vi "StandAlone_TransientDataCollection_Overhaul.vi"(8 "error in":errorcluster, 11 "Oscilloscope Configuration Array":T2(array[cluster]) {"vertical coupling" items=["AC", "DC", "Ground"]}) -> (0 "error out":errorcluster)   [LabVIEW 2019]
uses:
  <instrlib>/niScope/Controls/niScope vertical coupling.ctl
  <vilib>/Utility/file.llb/Write Delimited Spreadsheet (string).vi
  <instrlib>/niScope/Configure/Trigger/niScope Configure Trigger Software.vi
  <instrlib>/niScope/Acquire/Fetch/niScope Multi Fetch Binary 16.vi
panel:
  out "Sample Rate IND 2":dbl
  in  "stop 2":bool
  in  "Plot Data?":bool
  in  "numSamples":i32=-1
  in  "ON/OFF":bool
  in  "Using an RF Source?":bool
  in  "power (dBm)":dbl
  in  "frequency (GHz)":dbl
  in  "Apply RF Source Changes":bool
  in  "RF Source":refnum<visa-resource-name>
  out "current limit ind":dbl
  out "Channel 0 Reference Values":dbl[](array[numeric])
  out "CHANNEL 7 NAME":string
  out "CHANNEL 6 NAME":string
  out "CHANNEL 5 NAME":string
  out "CHANNEL 4 NAME":string
  out "CHANNEL 3 NAME":string
  out "CHANNEL 2 NAME":string
  out "CHANNEL 1 NAME":string
  out "CHANNEL 0 NAME":string
  out "RUN_FOLDER":path
  out "RESTART PROGRAM SOON (DATACOLLECT)":bool
  out "Sample Rate IND":dbl
  out "Channel To Mitigate (0-7) IND":i32
  out "Collecting Data":bool
  out "RESTART PROGRAM SOON (DATASTORE)":bool
  out "Threshold Value":dbl
  out "Num Loop 4 Reset Graph":i32
  out "Channel Graph Cumulative 7":dbl[](graph)
  out "Channel Graph Cumulative 6":dbl[](graph)
  out "Channel Graph Cumulative 5":dbl[](graph)
  out "Channel Graph Cumulative 4":dbl[](graph)
  out "Channel Graph Cumulative 3":dbl[](graph)
  out "Channel Graph Cumulative 2":dbl[](graph)
  out "Channel Graph Cumulative 1":dbl[](graph)
  out "Channel Graph Cumulative 0":dbl[](graph)
  out "Channel Graph 7":dbl[](graph)
  out "Channel Graph 6":dbl[](graph)
  out "Channel Graph 5":dbl[](graph)
  out "Channel Graph 4":dbl[](graph)
  out "Channel Graph 3":dbl[](graph)
  out "Channel Graph 2":dbl[](graph)
  out "Channel Graph 1":dbl[](graph)
  out "Channel Graph 0":dbl[](graph)
  in  "Channel To Mitigate (0-7)":i32
  out "Last Point Fetched":i32
  out "Total Points Fetched":i32
  out "NUMBER SAMPLES":i32
  out "XINC":dbl
  out "Nominal Current IND":dbl
  out "Percent Threshold IND":dbl
  out "EXCEED THRESHOLD":bool
  out "EXCEED DURATION":bool
  out "Over Threshold Number":i32
  out "number of resets":i32
  out "ENABLE STATE":bool
  in  "DC Power On":bool
  in  "TRANSIENT TIME DURATION (ms)":dbl=500.0
  in  "milliseconds to wait":u32
  in  "vertical coupling":T1=1 items=["AC", "DC", "Ground"]
  in  "min record length":i32=100000
  in  "INTIALIZE SCOPE":bool
  in  "50 ohm vertical range (V)":dbl=10.0 caption="50 ohm vertical range" format="%.2f"
  in  "Channel 0 50 ohms?":bool
  out "wfm info IND":T3(array[cluster]) caption="wfm info" {"reserved2" format="%.2f"; "reserved1" format="%.2f"; "offset" format="%^.3e"; "gain" format="%^.3e"; "xIncrement" format="%^.3e"; "relativeInitialX" format="%^.3e"; "absoluteInitialX" format="%^.3e"}
  out "AUTOMITIGATION ENABLED IND":bool
  in  "AUTOMITIGATION ENABLED":bool
  out "Vertical Range (V) IND":dbl=30.0 caption="Vertical Range (V)" format="%_3g"
  out "channels IND":string="0" caption="channels"
  out "Min. Sample Rate IND":dbl=50000.0 caption="Min. Sample Rate" format="%#_6p"
  in  "Ion (ex. Kr)":string
  in  "Effective LET":string
  in  "Board Number":string
  in  "DUT":string
  in  "Beam On?":bool
  in  "Percent Threshold":dbl
  in  "Nominal Mitigation Value":dbl
  out "Number Of Channels":i32
  in  "Plot Data?":bool=TRUE
  out "CURRENTPATH":path
  out "FOLDERCREATED":bool=TRUE
  out "IndicatorOutputs":cluster{"Run Information":string, string}
  out "Latchup_or_Transient":bool
  out "BinaryRefObjects":T4
  out "OscopeParamPath":path
  out "INITIALIZED":bool
  in  "APPLYPATH":bool
  in  "INPUTPATH":path=path "C:/Campaigns/LBNL_May_2025"
  in  "Max Points per Fetch":i32=-1
  in  "channels":string="Current,Vin,Vout1,Vout2,PowerGood1_2,EN1,EN2,BeamSignal" caption="channels (comma separated)"
  in  "Oscilloscope":refnum<k15>="PXIe-5172"
  in  "Min. Sample Rate":dbl=50000.0 format="%#_6p"
  in  "Vertical Range (V)":dbl=30.0 format="%_3g"
  out "RECORDING DATA":bool
  in  "BEGIN RECORDING":bool
  out "Present Mitigation Information":string
  out "NIDCPOWER_VOLT_CONF":dbl caption="voltage level IND" format="%.6p"
  out "NIDCPOWER_CHAN_CONF":string
  in  "NIDCPOWER_VOLT":dbl caption="voltage level" format="%.6p"
  in  "NIDCPOWER_CHAN":string="0"
  in  "resource name":refnum<k15>="Slot_4_PXIe4139" caption="DC Power PSU"
  in  "CHANGE MITIGATION":bool
  in  "Mitigation":u16(ring) items=["None", "Hardware", "PowerCycle", "EnableCircuit"]
  out "FINISH PROGRAM":bool
  in  "FORCED RESET":bool
  out "POWER STATE":bool
  in  "Channels to Parallelize (if selected)":u16(ring) items=["I1+I2", "ALL", "I2+I3"]
  out "Present Channel Configuration":string
  out "Channels Configured and Values":string[][](array[string])
  in  "Combination":u16(ring) items=["OFF", "SERIES", "PARALLEL"]
  in  "PSU":refnum<visa-resource-name>="USB0::0x05E6::0x2230::802901012767010005::INSTR"
  in  "Current Limit Channel 3":dbl
  in  "Current Limit Channel 2":dbl
  in  "Current Limit Channel 1":dbl
  in  "Voltage Channel 3":dbl
  in  "Voltage Channel 2":dbl
  in  "Voltage Channel 1":dbl
  in  "stop":bool
  in  "APPLY POWER SETTINGS":bool
  in  "POWER ON":bool
  # "11 In order, name all of the channels 0-7"
  # "3 press the white arrow"
  # "10 this is the maximum. Make it smaller for better resolution"
  # "OSCILLOSCOPE BLOCK"
  # "DATA BLOCK"
  # "5 enter where the data"
  # "Use this for step three"
  # "9 if needed"
  # "12 set the scope to the configurations from steps 9-11 on device"
  # "Nothing behind here"
  # "6 enter in values before each run"
  # "need to fix this"
  # "13,16 begin recording data"
  # "1"
  # "17 end program"
  # "2"
  # "14,15 saying the beam is on or could just have the TTL logic"
  # "7 enter in values before each run"
  # "POWER BLOCK"
  # "NI DCPower"
  # "NOTE THAT VISA POWER HAS THE NI DC POWER TURN OFF AS WELL"
  # "4"
  # "Current"
  # "8 power on device"
  # "Ignore all of this"
  # "7 power on device"
  # "7 power on device"
  # "7 power on device"
  # "7 power on device"
  # "7 power on device"
  # "7 power on device"
  # "7 power on device"
  # "7 power on device"
  # "7 power on device"
  # "7 power on device"
  # "7 power on device"
  # "7 power on device"
types:
  T1 = typedef "niScope vertical coupling.ctl" = i32
  T2 = cluster{"instrument handle out":refnum<k15>, string[], string[], "vertical range":dbl, "vertical coupling":T1, "Channel 0 50 ohms?":bool, "50 ohm vertical range (V)":dbl, "min record length":i32, "Actual Sample Rate":dbl, "channel names list":string}[]
  T3 = cluster{"actualSamples":i32, "absoluteInitialX":dbl, "relativeInitialX":dbl, "xIncrement":dbl, "offset":dbl, "gain":dbl, "reserved1":dbl, "reserved2":dbl}[]
  T4 = cluster{"appended path":path, "refnum out":refnum<file>, "refnum out":refnum<file>, "refnum out":refnum<file>}
  T5 = cluster{dbl[], dbl[], dbl[], dbl[], dbl[], dbl[], dbl[], dbl[]}
  T6 = cluster{"instrument handle out":refnum<k15>, string[], string[], "vertical range":dbl, "vertical coupling":T1, "Channel 0 50 ohms?":bool, "50 ohm vertical range (V)":dbl, "min record length":i32, "Actual Sample Rate":dbl, "channel names list":string}
  T7 = cluster{"array":dbl[], "array":dbl[], "array":dbl[], "array":dbl[], "array":dbl[], "array":dbl[], "array":dbl[], "array":dbl[]}
  T8 = cluster{"wfm info":cluster{"actualSamples":i32, "absoluteInitialX":dbl, "relativeInitialX":dbl, "xIncrement":dbl, "offset":dbl, "gain":dbl, "reserved1":dbl, "reserved2":dbl}[], "wfm":i16[][], "Beam On?":bool, i32}
  T9 = enum16{"open", "replace", "create", "open or create", "replace or create", "replace or create with confirmation"}
  T10 = enum16{"big-endian, network order", "native, host order", "little-endian"}
  T11 = cluster{"wfm info":cluster{"actualSamples":i32, "absoluteInitialX":dbl, "relativeInitialX":dbl, "xIncrement":dbl, "offset":dbl, "gain":dbl, "reserved1":dbl, "reserved2":dbl}[], "wfm":i16[][]}
  T12 = cluster{"actualSamples":i32, "absoluteInitialX":dbl, "relativeInitialX":dbl, "xIncrement":dbl, "offset":dbl, "gain":dbl, "reserved1":dbl, "reserved2":dbl}
  T13 = cluster{"AUTOMITIGATION ENABLED IND":bool, "Present Mitigation Information":string}
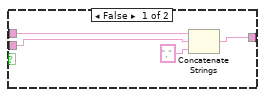
[diagram p2: hidden frame]
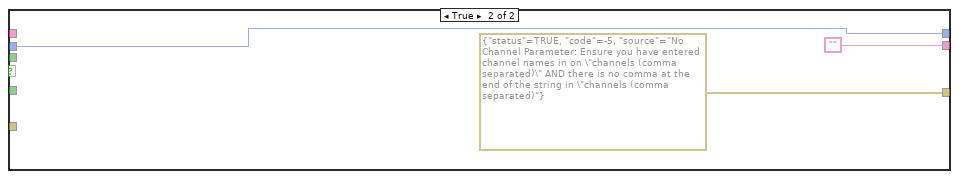
[diagram p3: hidden frame]
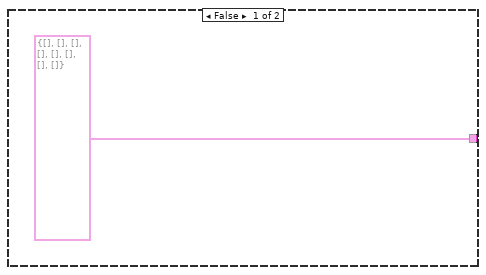
[diagram p6: hidden frame]
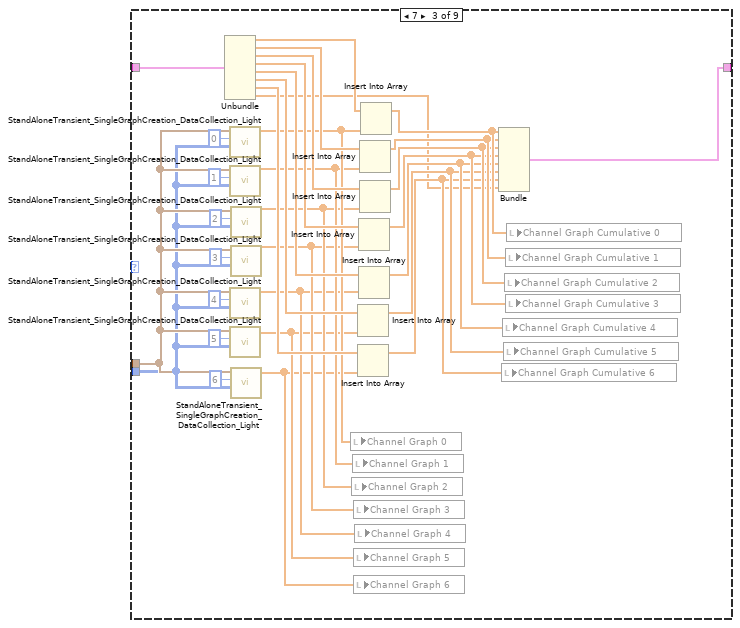
[diagram p8: hidden frame]
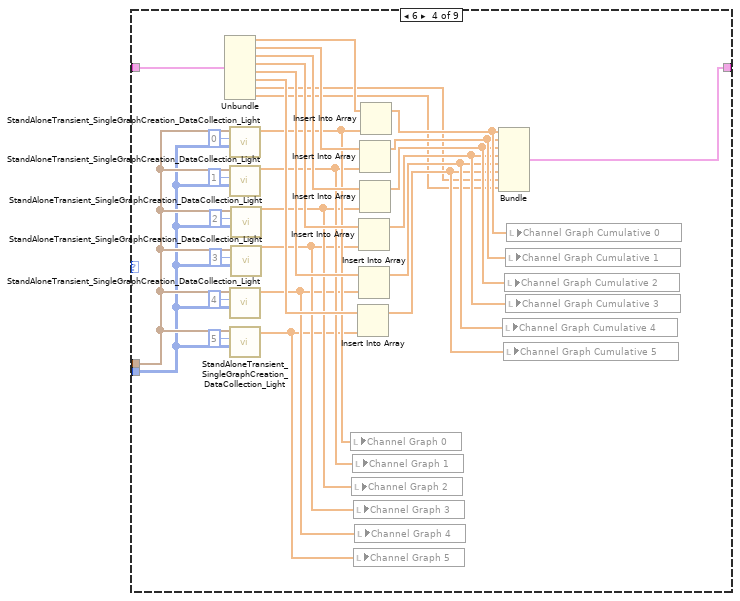
[diagram p9: hidden frame]
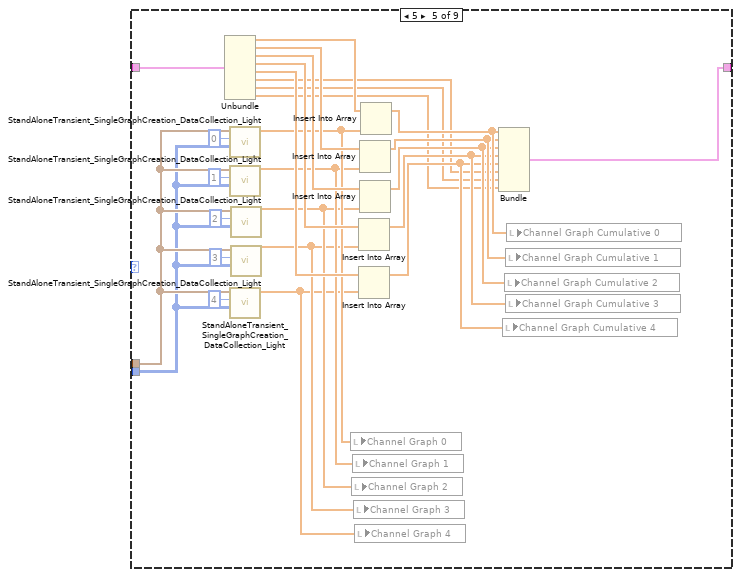
[diagram p10: hidden frame]
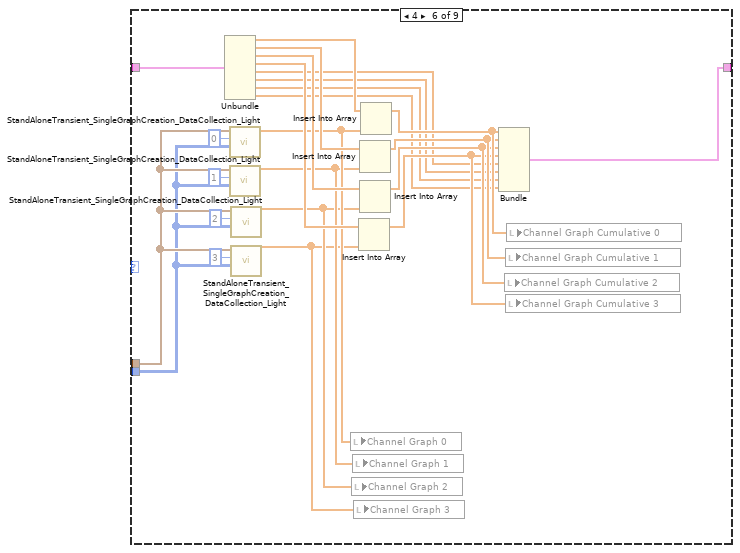
[diagram p11: hidden frame]
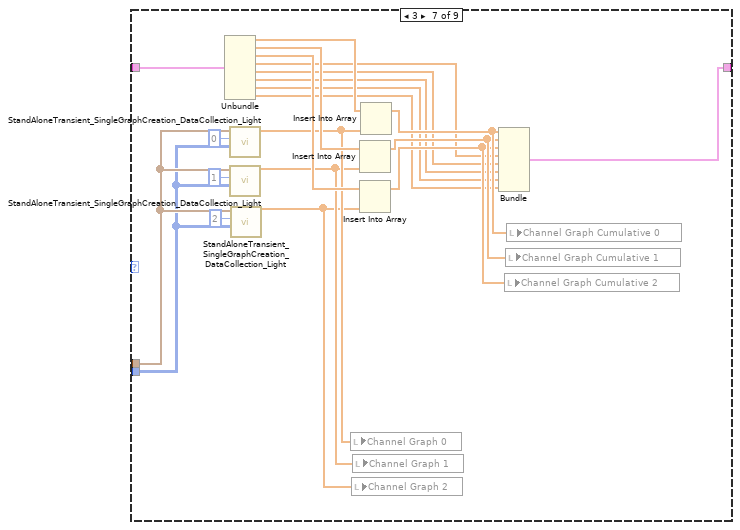
[diagram p12: hidden frame]
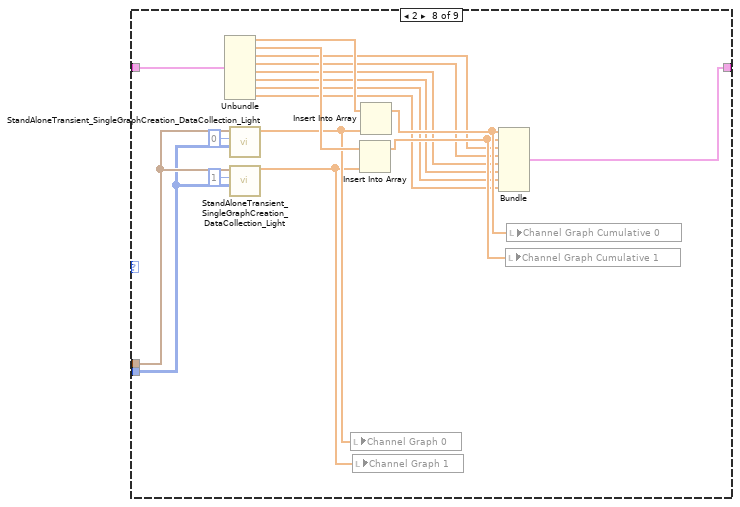
[diagram p13: hidden frame]
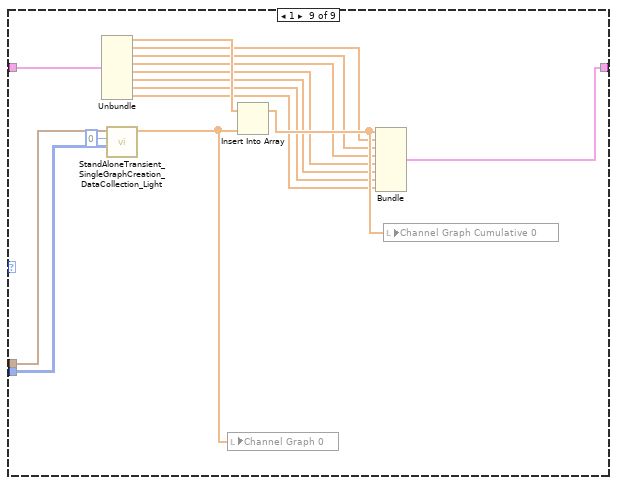
[diagram p14: hidden frame]
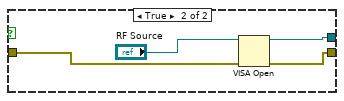
[diagram p16: hidden frame]
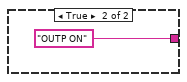
[diagram p18: hidden frame]
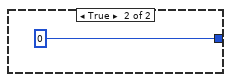
[diagram p19: hidden frame]
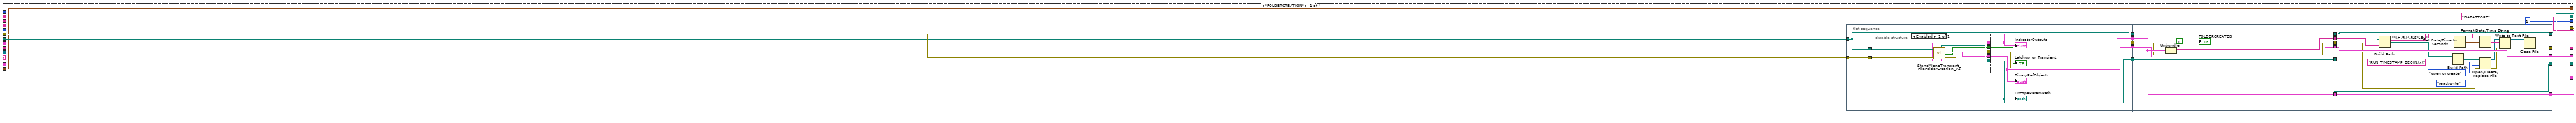
[diagram p20: hidden frame]
diagram:
  n1 = disable-structure shown="Disabled" {
    frame Disabled {
      n2 = Index Array(array="Oscilloscope Configuration Array", index=0) -> (element=w13:T6)
      n3 = Unbundle(w13) -> ("instrument handle out"=w7:refnum<k15>, w10:string[], "channel names list"=w12:string)  [unwired: 7 out]
      n4 = Array Size(array=w10) -> (size(s)=w9:i32)
      n5 = call <instrlib>:"niScope Initiate Acquisition.vi"("instrument handle"=w7, "error in"="error in") -> ("instrument handle out"=w5:refnum<k15>, "error out"=w6:errorcluster)  [unwired: 12 in]
      n6 = disable-structure shown="Disabled" {
        frame Disabled {
          n7 = flat-sequence {
            tunnel: _ -> [w29]
            tunnel: _ -> [w30]
            tunnel: _ -> [w31]
            tunnel: _ -> [w26]
            tunnel: _ -> [w32]
            tunnel: _ -> [w24]
            tunnel: _ -> [w33]
            tunnel: [w33] -> w22
            tunnel: [w23] -> w21
            tunnel: [w32] -> w20
            tunnel: [w25] -> w19
            tunnel: [w31] -> w18
            tunnel: [w30] -> w17
            tunnel: [w29] -> w16
            tunnel: [w118] -> _
            tunnel: [w117] -> _
            tunnel: ["WAIT4FOLDER"] -> _
            tunnel: _ -> [w100]
            tunnel: _ -> [w93]
            tunnel: [w91] -> _
            tunnel: w22 -> [w116]
            tunnel: w21 -> [w115]
            tunnel: w20 -> [w114]
            tunnel: w19 -> [w90]
            tunnel: w18 -> [w99]
            tunnel: w17 -> [w98]
            tunnel: w16 -> [w92]
            tunnel: [w90] -> _
            frame #0 {
              n8 = while {
                shift-right: [w49] -> _
                shift-left: w26 -> [w50]
                shift-right: [w35] -> _
                shift-left: 0 -> [w41]
                shift-right: [w43] -> w25
                shift-left: "" -> [w39]
                tunnel: [w49] -> _ mode=indexing
                tunnel: w24 -> [w38]
                tunnel: [w37] -> w23
                i -> [w48]
                stop <- w47 stop-if-true
                n9 = flat-sequence {
                  tunnel: w50 -> [w60]
                  tunnel: w48 -> [_]
                  tunnel: [w58] -> w46
                  tunnel: [w51] -> w45
                  tunnel: [w52] -> w44
                  tunnel: [w57] -> w42
                  tunnel: w41 -> [w57]
                  tunnel: [w56] -> w40
                  tunnel: w39 -> [w56]
                  tunnel: [w51] -> w34
                  tunnel: w46 -> [w72]
                  tunnel: w45 -> [w63]
                  tunnel: w44 -> [w71]
                  tunnel: w42 -> [w69]
                  tunnel: w40 -> [w68]
                  tunnel: w38 -> [w67]
                  tunnel: [w72] -> w49
                  tunnel: [w63] -> w47
                  tunnel: [w70] -> w43
                  tunnel: [w66] -> w37
                  tunnel: [w65] -> w36
                  tunnel: w34 -> [w64]
                  frame #0 {
                    n10 = Match Pattern(string=w60, regular expression=",") -> (before substring=w55:string, after substring=w58:string, offset past match=w62:i32)  [unwired: 1 in, 1 out]
                    n11 = Equal?(x=w55, y="") -> (x = y?=w53:bool)
                    n12 = Equal?(x=w62, y=-1) -> (x = y?=w51:bool)
                    n13 = And(x=w51, y=w53) -> (x .and. y?=w52:bool)
                  }
                  frame #1 {
                    n14 = case shown="False" w71 {
                      tunnel: [w73 ""] -> w70
                      tunnel: w69 -> [w78 w87]
                      tunnel: w68 -> [w76 _]
                      tunnel: [w78 w87] -> w65
                      tunnel: w67 -> [w77 _]
                      tunnel: [w77 errorcluster {"status"=TRUE, "code"=-5, "source"="No Channel Parameter: Ensure you have entered channel names in on \"channels (comma separated)\" AND there is no comma at the end of the string in \"channels (comma separated)"} ("error out")] -> w66
                      tunnel: w64 -> [_ _]
                      tunnel: w63 -> [w74 _]
                      frame False {
                        n15 = Number To Decimal String(number=w78) -> (decimal integer string=w75:string)  [unwired: 1 in]
                        n16 = case shown="True" w74 {
                          tunnel: w76 -> [w82 w85]
                          tunnel: w75 -> [w81 w84]
                          tunnel: [w79 w83] -> w73
                          frame False {
                            n17 = Concatenate Strings(w82, w81, "," ("string")) -> (w79:string)
                          }
                          frame True {
                            n18 = Concatenate Strings(w85, w84) -> (w83:string)
                          }
                        }
                      }
                      frame True {
                      }
                    }
                  }
                }
                n19 = Increment(x=w36) -> (x+1=w35:i32)
              }
            }
            frame #1 {
              w119 = u32 0 items=["1 mega ohm"=0, "50 ohms"=2] ("input impedance")
              w124 = 388 items=["Start"=482, "Trigger"=483, "Pretrigger"=477, "Now"=481, "Read Pointer"=388] ("Fetch:Fetch Relative To")
              # "3"
              n20 = String Length(string=w90) -> (length=w112:i32)
              n21 = Match Pattern(string=w90, regular expression="0") -> (offset past match=w102:i32)  [unwired: 1 in, 3 out]
              n22 = call <instrlib>:"niScope Configure Vertical.vi"("instrument handle"=w116, "vertical coupling"=w98, "channels"=w90, "vertical range"=w114, "error in"=w115) -> ("instrument handle out"=w121:refnum<k15>, "error out"=w120:errorcluster)  [unwired: 9 in]
              n23 = Quotient & Remainder(x=w112, y=2) -> (x-y*floor(x/y)=w109:i32, floor(x/y)=w110:i32)
              n24 = Not Equal?(x=w102, y=-1) -> (x != y?=w103:bool)
              n25 = And(x=w99, y=w103) -> (x .and. y?=w104:bool)
              n26 = Add(x=w109, y=w110) -> (x+y=w91:i32)
              n27 = call <instrlib>:"niScope Configure Chan Characteristics.vi"("instrument handle"=w121, "channels"=w90, "input impedance"=w119, "maximum input frequency"=0.0, "error in"=w120) -> ("instrument handle out"=w107:refnum<k15>, "error out"=w106:errorcluster)  [unwired: 9 in]
              n28 = case shown="True" w104 {
                tunnel: [w128 w138] -> w97
                tunnel: [w127 w137] -> w96
                tunnel: w107 -> [w128 w132]
                tunnel: w106 -> [w127 w131]
                tunnel: w100 -> [_ w129]
                frame False {
                }
                frame True {
                  w135 = u32 2 items=["1 mega ohm"=0, "50 ohms"=2] ("input impedance")
                  w130 = "0" ("channels")
                  n29 = call <instrlib>:"niScope Configure Vertical.vi"("instrument handle"=w132, "channels"=w130, "vertical range"=w129, "error in"=w131) -> ("instrument handle out"=w134:refnum<k15>, "error out"=w133:errorcluster)  [unwired: 10 in]
                  n30 = call <instrlib>:"niScope Configure Chan Characteristics.vi"("instrument handle"=w134, "channels"=w130, "input impedance"=w135, "maximum input frequency"=0.0, "error in"=w133) -> ("instrument handle out"=w138:refnum<k15>, "error out"=w137:errorcluster)  [unwired: 9 in]
                }
              }
              n31 = call <instrlib>:"niScope Configure Horizontal Timing.vi"("instrument handle"=w97, "min sample rate"=w92, "error in"=w96, "min record length"=w93) -> ("instrument handle out"=w94:refnum<k15>, "error out"=w95:errorcluster)  [unwired: 10 in]
              n32 = call-poly <instrlib>:"niScope Configure Trigger (poly).vi"("instrument handle"=w94, "error in"=w95) -> ("instrument handle out"=w123:refnum<k15>, "error out"=w122:errorcluster)  [unwired: 12 in]
              n33 = call <instrlib>:"niScope Initiate Acquisition.vi"("instrument handle"=w123, "error in"=w122) -> ("instrument handle out"=w125:refnum<k15>, "error out"=w126:errorcluster)  [unwired: 12 in]
              n34 = property class="niScope" props=["Fetch:Fetch Relative To", "Acquisition:Binary Sample Width", "Actual Sample Rate", "Actual Record Length"](reference=w125, error in=w126, "Fetch:Fetch Relative To"=w124) -> (reference out=w118:refnum<k15>, error out=w117:errorcluster, "Actual Sample Rate"=→"Sample Rate IND 2":dbl)  [unwired: 2 out]
            }
          }
        }
        frame Enabled {
        }
      }
      n35 = while {
        shift-right: [w148] -> w4
        shift-left: w6 -> [w158]
        tunnel: w5 -> [w157]
        tunnel: w12 -> [w156]
        tunnel: "numSamples" -> [w155]
        tunnel: w9 -> [w154]
        shift-right: [w151] -> _
        shift-left: _ -> [w150]
        tunnel: [w146] -> w3
        shift-right: [w139] -> _
        shift-left: 0 -> [w142]
        stop <- w147 stop-if-true
        n36 = Increment(x=w142) -> (x+1=w139:i32)
        n37 = Greater?(x=w139, y=1000000) -> (0:w143:bool)
        n38 = Not(x=w143) -> (.not. x?=w145:bool)
        n39 = call-poly <instrlib>:"niScope Fetch (poly).vi"("timeout"=0.0, "error in"=w158, "numSamples"=w155, "channels"=w156, "instrument handle"=w157) -> ("error out"=w148:errorcluster, "wfm"=w152:i16[][], "wfm info"=w153:T3, "instrument handle out"=w146:refnum<k15>)  [unwired: 3 in]
        n40 = Or(x="Plot Data?", y=w145) -> (x .or. y?=w140:bool)
        n41 = case shown="True" w140 {
          tunnel: w154 -> [_ w165]
          tunnel: w153 -> [_ w164]
          tunnel: w152 -> [_ w163]
          tunnel: [T5 {[], [], [], [], [], [], [], []} w162] -> w151
          tunnel: w150 -> [_ w161]
          frame False {
          }
          frame True {
            n42 = case shown="8" w165 {
              tunnel: w164 -> [_ w201 w234 w264 w291 w315 w336 w354 w369]
              tunnel: w163 -> [_ w200 w233 w263 w290 w314 w335 w353 w368]
              tunnel: [w166 w192 w203 w237 w266 w293 w318 w340 w359] -> w162
              tunnel: w161 -> [w166 w191 w226 w257 w285 w310 w332 w351 w367]
              frame 0, Default {
              }
              frame 8 {
                n43 = Unbundle(w191) -> (w183:dbl[], w184:dbl[], w185:dbl[], w186:dbl[], w187:dbl[], w188:dbl[], w189:dbl[], w190:dbl[])
                n44 = call "StandAloneTransient_SingleGraphCreation_DataCollection_Light.vi"("wfm"=w200, "index"=0, "wfm info"=w201) -> ("Array"=w182:dbl[])  [unwired: 8 in]
                n45 = call "StandAloneTransient_SingleGraphCreation_DataCollection_Light.vi"("wfm"=w200, "index"=1, "wfm info"=w201) -> ("Array"=w181:dbl[])  [unwired: 8 in]
                n46 = call "StandAloneTransient_SingleGraphCreation_DataCollection_Light.vi"("wfm"=w200, "index"=4, "wfm info"=w201) -> ("Array"=w178:dbl[])  [unwired: 8 in]
                n47 = call "StandAloneTransient_SingleGraphCreation_DataCollection_Light.vi"("wfm"=w200, "index"=5, "wfm info"=w201) -> ("Array"=w177:dbl[])  [unwired: 8 in]
                n48 = call "StandAloneTransient_SingleGraphCreation_DataCollection_Light.vi"("wfm"=w200, "index"=2, "wfm info"=w201) -> ("Array"=w180:dbl[])  [unwired: 8 in]
                n49 = call "StandAloneTransient_SingleGraphCreation_DataCollection_Light.vi"("wfm"=w200, "index"=3, "wfm info"=w201) -> ("Array"=w179:dbl[])  [unwired: 8 in]
                n50 = call "StandAloneTransient_SingleGraphCreation_DataCollection_Light.vi"("wfm"=w200, "index"=6, "wfm info"=w201) -> ("Array"=w176:dbl[])  [unwired: 8 in]
                n51 = call "StandAloneTransient_SingleGraphCreation_DataCollection_Light.vi"("wfm"=w200, "index"=7, "wfm info"=w201) -> ("Array"=w175:dbl[])  [unwired: 8 in]
                n52 = local write "Channel Graph 0"(w182) -> ()
                n53 = local write "Channel Graph 2"(w180) -> ()
                n54 = local write "Channel Graph 1"(w181) -> ()
                n55 = local write "Channel Graph 3"(w179) -> ()
                n56 = local write "Channel Graph 5"(w177) -> ()
                n57 = local write "Channel Graph 6"(w176) -> ()
                n58 = local write "Channel Graph 7"(w175) -> ()
                n59 = local write "Channel Graph 4"(w178) -> ()
                n60 = Insert Into Array(array=w190, new element=w175) -> (w167:dbl[])  [unwired: 1 in]
                n61 = Insert Into Array(array=w188, new element=w177) -> (w169:dbl[])  [unwired: 1 in]
                n62 = Insert Into Array(array=w189, new element=w176) -> (w168:dbl[])  [unwired: 1 in]
                n63 = Insert Into Array(array=w186, new element=w179) -> (w171:dbl[])  [unwired: 1 in]
                n64 = Insert Into Array(array=w187, new element=w178) -> (w170:dbl[])  [unwired: 1 in]
                n65 = Insert Into Array(array=w184, new element=w181) -> (w173:dbl[])  [unwired: 1 in]
                n66 = Insert Into Array(array=w185, new element=w180) -> (w172:dbl[])  [unwired: 1 in]
                n67 = Insert Into Array(array=w183, new element=w182) -> (w174:dbl[])  [unwired: 1 in]
                n68 = Bundle(w174, w173, w172, w171, w170, w169, w168, w167) -> (w192:T5)  [unwired: 1 in]
                n69 = local write "Channel Graph Cumulative 6"(w168) -> ()
                n70 = local write "Channel Graph Cumulative 4"(w170) -> ()
                n71 = local write "Channel Graph Cumulative 5"(w169) -> ()
                n72 = local write "Channel Graph Cumulative 7"(w167) -> ()
                n73 = local write "Channel Graph Cumulative 2"(w172) -> ()
                n74 = local write "Channel Graph Cumulative 1"(w173) -> ()
                n75 = local write "Channel Graph Cumulative 3"(w171) -> ()
                n76 = local write "Channel Graph Cumulative 0"(w174) -> ()
              }
              frame 7 {
                n77 = Unbundle(w226) -> (w219:dbl[], w220:dbl[], w221:dbl[], w222:dbl[], w223:dbl[], w224:dbl[], w225:dbl[], w204:dbl[])
                n78 = call "StandAloneTransient_SingleGraphCreation_DataCollection_Light.vi"("wfm"=w233, "index"=0, "wfm info"=w234) -> ("Array"=w218:dbl[])  [unwired: 8 in]
                n79 = call "StandAloneTransient_SingleGraphCreation_DataCollection_Light.vi"("wfm"=w233, "index"=1, "wfm info"=w234) -> ("Array"=w217:dbl[])  [unwired: 8 in]
                n80 = call "StandAloneTransient_SingleGraphCreation_DataCollection_Light.vi"("wfm"=w233, "index"=4, "wfm info"=w234) -> ("Array"=w214:dbl[])  [unwired: 8 in]
                n81 = call "StandAloneTransient_SingleGraphCreation_DataCollection_Light.vi"("wfm"=w233, "index"=5, "wfm info"=w234) -> ("Array"=w213:dbl[])  [unwired: 8 in]
                n82 = call "StandAloneTransient_SingleGraphCreation_DataCollection_Light.vi"("wfm"=w233, "index"=2, "wfm info"=w234) -> ("Array"=w216:dbl[])  [unwired: 8 in]
                n83 = call "StandAloneTransient_SingleGraphCreation_DataCollection_Light.vi"("wfm"=w233, "index"=3, "wfm info"=w234) -> ("Array"=w215:dbl[])  [unwired: 8 in]
                n84 = call "StandAloneTransient_SingleGraphCreation_DataCollection_Light.vi"("wfm"=w233, "index"=6, "wfm info"=w234) -> ("Array"=w212:dbl[])  [unwired: 8 in]
                n85 = local write "Channel Graph 0"(w218) -> ()
                n86 = local write "Channel Graph 2"(w216) -> ()
                n87 = local write "Channel Graph 1"(w217) -> ()
                n88 = local write "Channel Graph 3"(w215) -> ()
                n89 = local write "Channel Graph 5"(w213) -> ()
                n90 = local write "Channel Graph 6"(w212) -> ()
                n91 = local write "Channel Graph 4"(w214) -> ()
                n92 = Insert Into Array(array=w224, new element=w213) -> (w206:dbl[])  [unwired: 1 in]
                n93 = Insert Into Array(array=w225, new element=w212) -> (w205:dbl[])  [unwired: 1 in]
                n94 = Insert Into Array(array=w222, new element=w215) -> (w208:dbl[])  [unwired: 1 in]
                n95 = Insert Into Array(array=w223, new element=w214) -> (w207:dbl[])  [unwired: 1 in]
                n96 = Insert Into Array(array=w220, new element=w217) -> (w210:dbl[])  [unwired: 1 in]
                n97 = Insert Into Array(array=w221, new element=w216) -> (w209:dbl[])  [unwired: 1 in]
                n98 = Insert Into Array(array=w219, new element=w218) -> (w211:dbl[])  [unwired: 1 in]
                n99 = Bundle(w211, w210, w209, w208, w207, w206, w205, w204) -> (w203:T5)  [unwired: 1 in]
                n100 = local write "Channel Graph Cumulative 6"(w205) -> ()
                n101 = local write "Channel Graph Cumulative 4"(w207) -> ()
                n102 = local write "Channel Graph Cumulative 5"(w206) -> ()
                n103 = local write "Channel Graph Cumulative 2"(w209) -> ()
                n104 = local write "Channel Graph Cumulative 1"(w210) -> ()
                n105 = local write "Channel Graph Cumulative 3"(w208) -> ()
                n106 = local write "Channel Graph Cumulative 0"(w211) -> ()
              }
              frame 6 {
                n107 = Unbundle(w257) -> (w251:dbl[], w252:dbl[], w253:dbl[], w254:dbl[], w255:dbl[], w256:dbl[], w236:dbl[], w238:dbl[])
                n108 = call "StandAloneTransient_SingleGraphCreation_DataCollection_Light.vi"("wfm"=w263, "index"=0, "wfm info"=w264) -> ("Array"=w250:dbl[])  [unwired: 8 in]
                n109 = call "StandAloneTransient_SingleGraphCreation_DataCollection_Light.vi"("wfm"=w263, "index"=1, "wfm info"=w264) -> ("Array"=w249:dbl[])  [unwired: 8 in]
                n110 = call "StandAloneTransient_SingleGraphCreation_DataCollection_Light.vi"("wfm"=w263, "index"=4, "wfm info"=w264) -> ("Array"=w246:dbl[])  [unwired: 8 in]
                n111 = call "StandAloneTransient_SingleGraphCreation_DataCollection_Light.vi"("wfm"=w263, "index"=5, "wfm info"=w264) -> ("Array"=w245:dbl[])  [unwired: 8 in]
                n112 = call "StandAloneTransient_SingleGraphCreation_DataCollection_Light.vi"("wfm"=w263, "index"=2, "wfm info"=w264) -> ("Array"=w248:dbl[])  [unwired: 8 in]
                n113 = call "StandAloneTransient_SingleGraphCreation_DataCollection_Light.vi"("wfm"=w263, "index"=3, "wfm info"=w264) -> ("Array"=w247:dbl[])  [unwired: 8 in]
                n114 = local write "Channel Graph 0"(w250) -> ()
                n115 = local write "Channel Graph 2"(w248) -> ()
                n116 = local write "Channel Graph 1"(w249) -> ()
                n117 = local write "Channel Graph 3"(w247) -> ()
                n118 = local write "Channel Graph 5"(w245) -> ()
                n119 = local write "Channel Graph 4"(w246) -> ()
                n120 = Insert Into Array(array=w256, new element=w245) -> (w239:dbl[])  [unwired: 1 in]
                n121 = Insert Into Array(array=w254, new element=w247) -> (w241:dbl[])  [unwired: 1 in]
                n122 = Insert Into Array(array=w255, new element=w246) -> (w240:dbl[])  [unwired: 1 in]
                n123 = Insert Into Array(array=w252, new element=w249) -> (w243:dbl[])  [unwired: 1 in]
                n124 = Insert Into Array(array=w253, new element=w248) -> (w242:dbl[])  [unwired: 1 in]
                n125 = Insert Into Array(array=w251, new element=w250) -> (w244:dbl[])  [unwired: 1 in]
                n126 = Bundle(w244, w243, w242, w241, w240, w239, w236, w238) -> (w237:T5)  [unwired: 1 in]
                n127 = local write "Channel Graph Cumulative 4"(w240) -> ()
                n128 = local write "Channel Graph Cumulative 5"(w239) -> ()
                n129 = local write "Channel Graph Cumulative 2"(w242) -> ()
                n130 = local write "Channel Graph Cumulative 1"(w243) -> ()
                n131 = local write "Channel Graph Cumulative 3"(w241) -> ()
                n132 = local write "Channel Graph Cumulative 0"(w244) -> ()
              }
              frame 5 {
                n133 = Unbundle(w285) -> (w280:dbl[], w281:dbl[], w282:dbl[], w283:dbl[], w284:dbl[], w267:dbl[], w268:dbl[], w269:dbl[])
                n134 = call "StandAloneTransient_SingleGraphCreation_DataCollection_Light.vi"("wfm"=w290, "index"=0, "wfm info"=w291) -> ("Array"=w279:dbl[])  [unwired: 8 in]
                n135 = call "StandAloneTransient_SingleGraphCreation_DataCollection_Light.vi"("wfm"=w290, "index"=1, "wfm info"=w291) -> ("Array"=w278:dbl[])  [unwired: 8 in]
                n136 = call "StandAloneTransient_SingleGraphCreation_DataCollection_Light.vi"("wfm"=w290, "index"=4, "wfm info"=w291) -> ("Array"=w275:dbl[])  [unwired: 8 in]
                n137 = call "StandAloneTransient_SingleGraphCreation_DataCollection_Light.vi"("wfm"=w290, "index"=2, "wfm info"=w291) -> ("Array"=w277:dbl[])  [unwired: 8 in]
                n138 = call "StandAloneTransient_SingleGraphCreation_DataCollection_Light.vi"("wfm"=w290, "index"=3, "wfm info"=w291) -> ("Array"=w276:dbl[])  [unwired: 8 in]
                n139 = local write "Channel Graph 0"(w279) -> ()
                n140 = local write "Channel Graph 2"(w277) -> ()
                n141 = local write "Channel Graph 1"(w278) -> ()
                n142 = local write "Channel Graph 3"(w276) -> ()
                n143 = local write "Channel Graph 4"(w275) -> ()
                n144 = Insert Into Array(array=w283, new element=w276) -> (w271:dbl[])  [unwired: 1 in]
                n145 = Insert Into Array(array=w284, new element=w275) -> (w270:dbl[])  [unwired: 1 in]
                n146 = Insert Into Array(array=w281, new element=w278) -> (w273:dbl[])  [unwired: 1 in]
                n147 = Insert Into Array(array=w282, new element=w277) -> (w272:dbl[])  [unwired: 1 in]
                n148 = Insert Into Array(array=w280, new element=w279) -> (w274:dbl[])  [unwired: 1 in]
                n149 = Bundle(w274, w273, w272, w271, w270, w267, w268, w269) -> (w266:T5)  [unwired: 1 in]
                n150 = local write "Channel Graph Cumulative 4"(w270) -> ()
                n151 = local write "Channel Graph Cumulative 2"(w272) -> ()
                n152 = local write "Channel Graph Cumulative 1"(w273) -> ()
                n153 = local write "Channel Graph Cumulative 3"(w271) -> ()
                n154 = local write "Channel Graph Cumulative 0"(w274) -> ()
              }
              frame 4 {
                n155 = Unbundle(w310) -> (w306:dbl[], w307:dbl[], w308:dbl[], w309:dbl[], w294:dbl[], w295:dbl[], w296:dbl[], w297:dbl[])
                n156 = call "StandAloneTransient_SingleGraphCreation_DataCollection_Light.vi"("wfm"=w314, "index"=0, "wfm info"=w315) -> ("Array"=w305:dbl[])  [unwired: 8 in]
                n157 = call "StandAloneTransient_SingleGraphCreation_DataCollection_Light.vi"("wfm"=w314, "index"=1, "wfm info"=w315) -> ("Array"=w304:dbl[])  [unwired: 8 in]
                n158 = call "StandAloneTransient_SingleGraphCreation_DataCollection_Light.vi"("wfm"=w314, "index"=2, "wfm info"=w315) -> ("Array"=w303:dbl[])  [unwired: 8 in]
                n159 = call "StandAloneTransient_SingleGraphCreation_DataCollection_Light.vi"("wfm"=w314, "index"=3, "wfm info"=w315) -> ("Array"=w302:dbl[])  [unwired: 8 in]
                n160 = local write "Channel Graph 0"(w305) -> ()
                n161 = local write "Channel Graph 2"(w303) -> ()
                n162 = local write "Channel Graph 1"(w304) -> ()
                n163 = local write "Channel Graph 3"(w302) -> ()
                n164 = Insert Into Array(array=w309, new element=w302) -> (w298:dbl[])  [unwired: 1 in]
                n165 = Insert Into Array(array=w307, new element=w304) -> (w300:dbl[])  [unwired: 1 in]
                n166 = Insert Into Array(array=w308, new element=w303) -> (w299:dbl[])  [unwired: 1 in]
                n167 = Insert Into Array(array=w306, new element=w305) -> (w301:dbl[])  [unwired: 1 in]
                n168 = Bundle(w301, w300, w299, w298, w294, w295, w296, w297) -> (w293:T5)  [unwired: 1 in]
                n169 = local write "Channel Graph Cumulative 2"(w299) -> ()
                n170 = local write "Channel Graph Cumulative 1"(w300) -> ()
                n171 = local write "Channel Graph Cumulative 3"(w298) -> ()
                n172 = local write "Channel Graph Cumulative 0"(w301) -> ()
              }
              frame 3 {
                n173 = Unbundle(w332) -> (w329:dbl[], w330:dbl[], w331:dbl[], w317:dbl[], w319:dbl[], w320:dbl[], w321:dbl[], w322:dbl[])
                n174 = call "StandAloneTransient_SingleGraphCreation_DataCollection_Light.vi"("wfm"=w335, "index"=0, "wfm info"=w336) -> ("Array"=w328:dbl[])  [unwired: 8 in]
                n175 = call "StandAloneTransient_SingleGraphCreation_DataCollection_Light.vi"("wfm"=w335, "index"=1, "wfm info"=w336) -> ("Array"=w327:dbl[])  [unwired: 8 in]
                n176 = call "StandAloneTransient_SingleGraphCreation_DataCollection_Light.vi"("wfm"=w335, "index"=2, "wfm info"=w336) -> ("Array"=w326:dbl[])  [unwired: 8 in]
                n177 = local write "Channel Graph 0"(w328) -> ()
                n178 = local write "Channel Graph 2"(w326) -> ()
                n179 = local write "Channel Graph 1"(w327) -> ()
                n180 = Insert Into Array(array=w330, new element=w327) -> (w324:dbl[])  [unwired: 1 in]
                n181 = Insert Into Array(array=w331, new element=w326) -> (w323:dbl[])  [unwired: 1 in]
                n182 = Insert Into Array(array=w329, new element=w328) -> (w325:dbl[])  [unwired: 1 in]
                n183 = Bundle(w325, w324, w323, w317, w319, w320, w321, w322) -> (w318:T5)  [unwired: 1 in]
                n184 = local write "Channel Graph Cumulative 2"(w323) -> ()
                n185 = local write "Channel Graph Cumulative 1"(w324) -> ()
                n186 = local write "Channel Graph Cumulative 0"(w325) -> ()
              }
              frame 2 {
                n187 = Unbundle(w351) -> (w349:dbl[], w350:dbl[], w338:dbl[], w339:dbl[], w341:dbl[], w342:dbl[], w343:dbl[], w344:dbl[])
                n188 = call "StandAloneTransient_SingleGraphCreation_DataCollection_Light.vi"("wfm"=w353, "index"=0, "wfm info"=w354) -> ("Array"=w348:dbl[])  [unwired: 8 in]
                n189 = call "StandAloneTransient_SingleGraphCreation_DataCollection_Light.vi"("wfm"=w353, "index"=1, "wfm info"=w354) -> ("Array"=w347:dbl[])  [unwired: 8 in]
                n190 = local write "Channel Graph 0"(w348) -> ()
                n191 = local write "Channel Graph 1"(w347) -> ()
                n192 = Insert Into Array(array=w350, new element=w347) -> (w345:dbl[])  [unwired: 1 in]
                n193 = Insert Into Array(array=w349, new element=w348) -> (w346:dbl[])  [unwired: 1 in]
                n194 = Bundle(w346, w345, w338, w339, w341, w342, w343, w344) -> (w340:T5)  [unwired: 1 in]
                n195 = local write "Channel Graph Cumulative 1"(w345) -> ()
                n196 = local write "Channel Graph Cumulative 0"(w346) -> ()
              }
              frame 1 {
                n197 = Unbundle(w367) -> (w366:dbl[], w356:dbl[], w357:dbl[], w358:dbl[], w360:dbl[], w361:dbl[], w362:dbl[], w363:dbl[])
                n198 = call "StandAloneTransient_SingleGraphCreation_DataCollection_Light.vi"("wfm"=w368, "index"=0, "wfm info"=w369) -> ("Array"=w365:dbl[])  [unwired: 8 in]
                n199 = local write "Channel Graph 0"(w365) -> ()
                n200 = Insert Into Array(array=w366, new element=w365) -> (w364:dbl[])  [unwired: 1 in]
                n201 = Bundle(w364, w356, w357, w358, w360, w361, w362, w363) -> (w359:T5)  [unwired: 1 in]
                n202 = local write "Channel Graph Cumulative 0"(w364) -> ()
              }
            }
          }
        }
        n203 = Or(x=w148, y="stop 2") -> (x .or. y?=w147:bool)
      }
      n204 = call <instrlib>:"niScope Abort.vi"("instrument handle"=w3, "error in"=w4) -> ("error out"=→"error out":errorcluster)  [unwired: 12 in, 1 out]
    }
    frame Enabled {
    }
  }
  n205 = disable-structure shown="Enabled" {
    frame Enabled {
      # "C:\\NULL"
      # "Moved Graph outputting into the collection to make it closer to live. Moved queueing to after the software reading as well so we can put everything inside the queueing element for better synchronization"
      # "Moved Software reading to the collection terminal to make the processing faster"
      n206 = flat-sequence {
        tunnel: [w380] -> w373
        tunnel: [w379] -> w372
        tunnel: w373 -> [w417]
        tunnel: w372 -> [w418]
        tunnel: [w386] -> w371
        frame #0 {
          w381 = FALSE  # Reset Device
          n207 = local write "number of resets"(0 ("number of resets")) -> ()
          n208 = local write "NIDCPOWER_VOLT_CONF"(0.0 ("NIDCPOWER_VOLT_CONF")) -> ()
          n209 = local write "Channel To Mitigate (0-7) IND"(0) -> ()
          n210 = local write "FINISH PROGRAM"(FALSE) -> ()
          n211 = local write "Collecting Data"(FALSE ("Collecting Data")) -> ()
          n212 = local write "EXCEED DURATION"(FALSE) -> ()
          n213 = local write "FOLDERCREATED"(FALSE) -> ()
          n214 = local write "NIDCPOWER_CHAN_CONF"("0" ("NIDCPOWER_CHAN_CONF")) -> ()
          n215 = call <instrlib>:"niScope Initialize.vi"("resource name"="Oscilloscope", "reset device"=w381) -> ("instrument handle"=w379:refnum<k15>, "error out"=w380:errorcluster)  [unwired: 12 in]
        }
        frame #1 {
          (unwired) T11 {"wfm info"=[], "wfm"=[]} ("cluster")
          # "OVERTHRESHOLD"
          # "INSIDE TRANSIENT"
          # "INITIAL TIME STAMP INSIDE TRANSIENT"
          # "TOTAL POINTS COLLECTED"
          # "INITIAL\nTIME\nSTAMP \nINSIDE \nTRANSIENT"
          # "INSIDE TRANSIENT"
          # "Capture Number"
          # "MAY WANT TO MAKE THE CONDITIONAL COMPONENT A SUBVI IN ITSELF"
          n216 = Obtain Queue(element data type=T8 {"wfm info"=[], "wfm"=[], "Beam On?"=FALSE, 0} ("cluster"), error in (no error)=w417) -> (queue out=w398:refnum<queue>, error out=w394:errorcluster)  [unwired: 3 in, 1 out]
          n217 = case shown="False" "Using an RF Source?" {
            tunnel: w394 -> [w427 w432]
            tunnel: [w427 w431] -> w393
            tunnel: [refnum<visa-resource-name> refnum ("RF Source") w429] -> w392
            frame False {
            }
            frame True {
              n218 = VISA Open(error in (no error)=w432, VISA resource name="RF Source") -> (VISA resource name=w429:refnum<visa-resource-name>, error out=w431:errorcluster)  [unwired: 3 in]
            }
          }
          n219 = while {
            shift-right: [w460] -> _
            shift-left: path "C:/NULL" ("base path") -> [w459]
            shift-right: [w458] -> _
            shift-left: "HOLDOFF" -> [w461]
            shift-right: [w457] -> w389
            shift-left: w393 -> [w437]
            shift-right: [w456] -> _
            shift-left: path "" ("OscopeParamPath") -> [w453]
            shift-right: [w455] -> _
            shift-left: T4 {"appended path"=path "", "refnum out"=refnum, "refnum out"=refnum, "refnum out"=refnum} ("BinaryRefObjects") -> [w452]
            shift-right: [w454] -> _
            shift-left: cluster{"name or relative path":string, string} {"name or relative path"="", ""} ("IndicatorOutputs") -> [w451]
            tunnel: w398 -> [w448]
            shift-right: [w449] -> _
            shift-left: 0 -> [w450]
            shift-right: [w442] -> _
            shift-left: T3 [] ("wfm info") -> [w443]
            tunnel: w392 -> [w435]
            tunnel: [w433] -> w387
            i -> [w439]
            stop <- w462 stop-if-true
            n220 = case shown="True" "Apply RF Source Changes" {
              tunnel: w437 -> [w464 w476]
              tunnel: [w464 w469] -> w436
              tunnel: w435 -> [w463 w475]
              tunnel: [w463 w467] -> w433
              frame False {
              }
              frame True {
                n221 = Multiply(x=1000000000.0 ("y"), y="frequency (GHz)") -> (x*y=w473:dbl)
                n222 = Number To Fractional String(number=w473) -> (F-format string=w484:string)  [unwired: 3 in]
                n223 = case shown="False" "ON/OFF" {
                  tunnel: ["OUTP OFF" ("write buffer") "OUTP ON" ("write buffer")] -> w471
                  frame False {
                  }
                  frame True {
                  }
                }
                n224 = Number To Fractional String(number="power (dBm)") -> (F-format string=w479:string)  [unwired: 3 in]
                n225 = Concatenate Strings("freq " ("string"), w484) -> (w483:string)
                n226 = Concatenate Strings("pow " ("string"), w479) -> (w481:string)
                n227 = VISA Write(VISA resource name=w475, write buffer=w483, error in (no error)=w476) -> (VISA resource name out=w480:refnum<visa-resource-name>, error out=w477:errorcluster)  [unwired: 1 out]
                n228 = VISA Write(VISA resource name=w480, write buffer=w481, error in (no error)=w477) -> (VISA resource name out=w468:refnum<visa-resource-name>, error out=w470:errorcluster)  [unwired: 1 out]
                n229 = VISA Write(VISA resource name=w468, write buffer=w471, error in (no error)=w470) -> (VISA resource name out=w467:refnum<visa-resource-name>, error out=w469:errorcluster)  [unwired: 1 out]
              }
            }
            n230 = Greater?(x=w439, y=2100000000) -> (0:w440:bool)
            n231 = case shown="False" w440 {
              tunnel: [w487 0] -> w438
              tunnel: w439 -> [w487 _]
              frame False {
              }
              frame True {
              }
            }
            n232 = case shown="\"DATASTORE\"" w461 {
              selector: w461 -> [_ w588 _ w966]
              tunnel: [w506 w599 w846 w969] -> w460
              tunnel: w459 -> [w508 w599 w846 w970]
              tunnel: ["DATASTORE" w587 w860 w967] -> w458
              tunnel: w436 -> [w509 w594 w845 w965]
              tunnel: [w489 w567 w856 w965] -> w457
              tunnel: [w504 w559 w858 w964] -> w456
              tunnel: [w502 w561 w861 w963] -> w455
              tunnel: [w500 w560 w847 w962] -> w454
              tunnel: w453 -> [_ w559 w858 w964]
              tunnel: w452 -> [_ w591 w861 w963]
              tunnel: w451 -> [_ w560 w847 w962]
              tunnel: w438 -> [_ w598 _ w956]
              tunnel: w450 -> [_ w597 w862 w961]
              tunnel: [1 w571 w862 w961] -> w449
              tunnel: w448 -> [_ w590 _ _]
              tunnel: "DUT" -> [_ _ w863 _]
              tunnel: "Board Number" -> [_ _ w864 _]
              tunnel: "Effective LET" -> [_ _ w866 _]
              tunnel: "Ion (ex. Kr)" -> [_ _ w865 _]
              tunnel: [w497 w557 w859 w960] -> w442
              tunnel: w443 -> [w497 w556 w859 w960]
              frame "FOLDERCREATION" {
                n233 = flat-sequence {
                  tunnel: w509 -> [w510]
                  tunnel: w508 -> [w516]
                  tunnel: [w516] -> w507
                  tunnel: [w515] -> w503
                  tunnel: [w514] -> w501
                  tunnel: [w512] -> w499
                  tunnel: [w511] -> w490
                  tunnel: w507 -> [w529]
                  tunnel: w503 -> [w528]
                  tunnel: w501 -> [w527]
                  tunnel: w499 -> [w526]
                  tunnel: [w529] -> w496
                  tunnel: [w528] -> w495
                  tunnel: [w527] -> w494
                  tunnel: [w526] -> w493
                  tunnel: [w525] -> w492
                  tunnel: [w524] -> w491
                  tunnel: w490 -> [w524]
                  tunnel: [w547] -> w500
                  tunnel: [w548] -> w502
                  tunnel: [w549] -> w504
                  tunnel: [w534] -> w506
                  tunnel: w496 -> [w534]
                  tunnel: w495 -> [w549]
                  tunnel: w494 -> [w548]
                  tunnel: w493 -> [w547]
                  tunnel: w492 -> [w533]
                  tunnel: [w532] -> w489
                  tunnel: w491 -> [w531]
                  frame #0 {
                    n234 = disable-structure shown="Enabled" {
                      disable-tunnel: w516 -> [w522]
                      disable-tunnel: [w521] -> w515
                      disable-tunnel: [w520] -> w514
                      disable-tunnel: [w519] -> w513
                      disable-tunnel: [w517] -> w512
                      disable-tunnel: [w518] -> w511
                      disable-tunnel: w510 -> [w523]
                      frame Enabled {
                        n235 = call "StandAloneTransient_FileFolderCreation_V2.vi"("error in (no error)"=w523, "base path"=w522) -> ("error out"=w518:errorcluster, "Latchup_or_Transient"=w519:bool, "BinaryRefObjects"=w520:T4, "IndicatorOutputs"=w517:cluster{"name or relative path":string, string}, "OscopeParamPath"=w521:path)  [unwired: 4 in, 1 out]
                      }
                    }
                    "OscopeParamPath" <- w515
                    "BinaryRefObjects" <- w514
                    "Latchup_or_Transient" <- w513
                    "IndicatorOutputs" <- w512
                  }
                  frame #1 {
                    n236 = Unbundle(w526) -> ("name or relative path"=w525:string)  [unwired: 1 out]
                    "FOLDERCREATED" <- TRUE
                  }
                  frame #2 {
                    n237 = Build Path(base path=w534, name or relative path=w533) -> (appended path=w546:path)
                    n238 = Build Path(base path=w546, name or relative path="RUN_TIMESTAMP_BEGIN.txt") -> (appended path=w541:path)
                    n239 = Get Date/Time In Seconds() -> (seconds since 1Jan1904=w544:timestamp)
                    n240 = Format Date/Time String(time format string (%c)="%H.%M.%S%8u", seconds (now)=w544) -> (date/time string=w545:string)  [unwired: 1 in]
                    n241 = Open/Create/Replace File(file path (use dialog)=w541, error in=w531, operation (0:open)=T9."open or create", access (0:read/write)=enum16{"read/write", "read-only", "write-only"}."read/write") -> (refnum out=w539:refnum<file>, error out=w540:errorcluster)  [unwired: 2 in, 1 out]
                    n242 = Write to Text File(file (use dialog)=w539, text=w545, error in=w540) -> (refnum out=w543:refnum<file>, error out=w542:errorcluster)  [unwired: 1 in, 1 out]
                    n243 = Close File(refnum=w543, error in=w542) -> (error out=w532:errorcluster)  [unwired: 1 out]
                  }
                }
              }
              frame "DATASTORE" {
                # "IMPEMENT THE ACTUAL DATASTORE USING THE ENQUEING THAT WE KNOW FROM OLD DATACOLLECTION VIS"
                n244 = flat-sequence {
                  tunnel: w598 -> [w600]
                  tunnel: w597 -> [w602]
                  tunnel: [w604] -> w596
                  tunnel: [w603] -> w595
                  tunnel: w594 -> [w603]
                  tunnel: [w602] -> w593
                  tunnel: [w601] -> w592
                  tunnel: w591 -> [w601]
                  tunnel: w596 -> [w619]
                  tunnel: w595 -> [w618]
                  tunnel: w593 -> [w616]
                  tunnel: w592 -> [w615]
                  tunnel: [w617] -> w555
                  tunnel: [w614] -> w554
                  tunnel: [w613] -> w553
                  tunnel: [w612] -> w552
                  tunnel: [w611] -> w551
                  tunnel: [w610] -> w550
                  tunnel: w590 -> [w705]
                  tunnel: [w700] -> w589
                  tunnel: [w698] -> w585
                  tunnel: [w696] -> w583
                  tunnel: [w695] -> w580
                  tunnel: [w694] -> w578
                  tunnel: [w693] -> w576
                  tunnel: [w692] -> w574
                  tunnel: [w691] -> w572
                  tunnel: [w690] -> w569
                  tunnel: w550 -> [w690]
                  tunnel: w551 -> [w691]
                  tunnel: w552 -> [w695]
                  tunnel: w553 -> [w694]
                  tunnel: w554 -> [w693]
                  tunnel: w555 -> [w704]
                  tunnel: w589 -> [w719]
                  tunnel: w588 -> [w718]
                  tunnel: [w717] -> w587
                  tunnel: [w716] -> w586
                  tunnel: w585 -> [w716]
                  tunnel: [TRUE] -> w584
                  tunnel: w583 -> [_]
                  tunnel: [w715] -> w582
                  tunnel: [w714] -> w581
                  tunnel: w580 -> [w714]
                  tunnel: [w713] -> w579
                  tunnel: w578 -> [w713]
                  tunnel: [w712] -> w577
                  tunnel: w576 -> [w712]
                  tunnel: [w711] -> w575
                  tunnel: w574 -> [w711]
                  tunnel: [w710] -> w573
                  tunnel: w572 -> [w710]
                  tunnel: [w709] -> w570
                  tunnel: w569 -> [w709]
                  tunnel: w586 -> [w736]
                  tunnel: w584 -> [w735]
                  tunnel: w582 -> [w734]
                  tunnel: w581 -> [w733]
                  tunnel: w579 -> [w731]
                  tunnel: w577 -> [w730]
                  tunnel: w575 -> [w732]
                  tunnel: w573 -> [w729]
                  tunnel: w570 -> [w724]
                  tunnel: [w729] -> w568
                  tunnel: [w728] -> w566
                  tunnel: [w727] -> w565
                  tunnel: [w726] -> w564
                  tunnel: [w725] -> w563
                  tunnel: [w724] -> w562
                  tunnel: w556 -> [w723]
                  tunnel: [w722] -> w558
                  tunnel: [w842] -> w571
                  tunnel: w568 -> [w842]
                  tunnel: [w841] -> w567
                  tunnel: w566 -> [w841]
                  tunnel: w565 -> [w840]
                  tunnel: w564 -> [w839]
                  tunnel: w563 -> [w838]
                  tunnel: w562 -> [w837]
                  tunnel: [w836] -> w561
                  tunnel: w558 -> [w835]
                  tunnel: [w835] -> w557
                  frame #0 {
                    # "Iterations of the buffer loop until the next file is made. Tradeoff: Larger = worry about overflow \nSmaller = smaller files to process and less likelihood of overflowing, but more to push through the reading code which is bottlenecked by the write to csv code"
                    n245 = Quotient & Remainder(x=w600, y=100) -> (x-y*floor(x/y)=w607:i32, floor(x/y)=w608:i32)
                    n246 = Equal To 0?(x=w607) -> (x = 0?=w605:bool)
                    n247 = Not Equal To 0?(x=w608) -> (x != 0?=w606:bool)
                    n248 = And(x=w605, y=w606) -> (x .and. y?=w604:bool)
                  }
                  frame #1 {
                    n249 = case shown="True" w619 {
                      tunnel: w618 -> [w626 w643]
                      tunnel: [w626 w630] -> w617
                      tunnel: w616 -> [w621 w642]
                      tunnel: w615 -> [w625 w641]
                      tunnel: [w622 w633] -> w614
                      tunnel: [w623 w632] -> w613
                      tunnel: [w624 w631] -> w612
                      tunnel: [w621 w629] -> w611
                      tunnel: [w620 w628] -> w610
                      frame False {
                        n250 = Unbundle(w625) -> ("appended path"=w620:path, "refnum out"=w624:refnum<file>, "refnum out"=w623:refnum<file>, "refnum out"=w622:refnum<file>)
                      }
                      frame True {
                        n251 = flat-sequence {
                          tunnel: w643 -> [w650]
                          tunnel: w642 -> [w666]
                          tunnel: w641 -> [w665]
                          tunnel: [w652] -> w640
                          tunnel: [w651] -> w639
                          tunnel: [w650] -> w638
                          tunnel: [w649] -> w637
                          tunnel: [w648] -> w636
                          tunnel: [w647] -> w635
                          tunnel: [w646] -> w634
                          tunnel: [w645] -> w629
                          tunnel: [w644] -> w627
                          tunnel: w640 -> [w687]
                          tunnel: w639 -> [w686]
                          tunnel: w638 -> [w681]
                          tunnel: w637 -> [w675]
                          tunnel: w636 -> [w674]
                          tunnel: w635 -> [w673]
                          tunnel: w634 -> [w672]
                          tunnel: [w671] -> w633
                          tunnel: [w670] -> w632
                          tunnel: [w669] -> w631
                          tunnel: [w668] -> w630
                          tunnel: [w667] -> w628
                          tunnel: w627 -> [w667]
                          frame #0 {
                            n252 = Increment(x=w666) -> (x+1=w645:i32)
                            n253 = Number To Decimal String(number=w645) -> (decimal integer string=w655:string)  [unwired: 1 in]
                            n254 = Number To Decimal String(number=w645) -> (decimal integer string=w658:string)  [unwired: 1 in]
                            n255 = Number To Decimal String(number=w645) -> (decimal integer string=w662:string)  [unwired: 1 in]
                            n256 = Concatenate Strings("SamplePerCap_", w655, ".sbdf" ("string")) -> (w653:string)
                            n257 = Concatenate Strings("WaveformData_", w658, ".sbdf" ("string")) -> (w657:string)
                            n258 = Concatenate Strings("SampleData_", w662, ".sbdf" ("string")) -> (w661:string)
                            n259 = Unbundle(w665) -> ("appended path"=w644:path, "refnum out"=w651:refnum<file>, "refnum out"=w647:refnum<file>, "refnum out"=w646:refnum<file>)
                            n260 = Build Path(base path=w644, name or relative path=w653) -> (appended path=w648:path)
                            n261 = Build Path(base path=w644, name or relative path=w657) -> (appended path=w649:path)
                            n262 = Build Path(base path=w644, name or relative path=w661) -> (appended path=w652:path)
                          }
                          frame #1 {
                            n263 = Close File(refnum=w686, error in=w681) -> (error out=w680:errorcluster)  [unwired: 1 out]
                            n264 = Open/Create/Replace File(file path (use dialog)=w687, error in=w680, operation (0:open)=T9."open or create", access (0:read/write)=enum16{"read/write", "read-only", "write-only"}."read/write") -> (refnum out=w669:refnum<file>, error out=w679:errorcluster)  [unwired: 2 in, 1 out]
                            n265 = Close File(refnum=w673, error in=w679) -> (error out=w678:errorcluster)  [unwired: 1 out]
                            n266 = Open/Create/Replace File(file path (use dialog)=w675, error in=w678, operation (0:open)=T9."open or create", access (0:read/write)=enum16{"read/write", "read-only", "write-only"}."read/write") -> (refnum out=w670:refnum<file>, error out=w677:errorcluster)  [unwired: 2 in, 1 out]
                            n267 = Close File(refnum=w672, error in=w677) -> (error out=w676:errorcluster)  [unwired: 1 out]
                            n268 = Open/Create/Replace File(file path (use dialog)=w674, error in=w676, operation (0:open)=T9."open or create", access (0:read/write)=enum16{"read/write", "read-only", "write-only"}."read/write") -> (refnum out=w671:refnum<file>, error out=w668:errorcluster)  [unwired: 2 in, 1 out]
                          }
                        }
                      }
                    }
                  }
                  frame #2 {
                    n269 = local read "RECORDING DATA"() -> (w703:bool)
                    n270 = Get Queue Status(queue=w705, error in (no error)=w704) -> (queue out=w706:refnum<queue>, error out=w699:errorcluster, # elements in queue=w697:i32)  [unwired: 1 in, 5 out]
                    n271 = Equal To 0?(x=w697) -> (x = 0?=w701:bool)
                    n272 = Greater Than 0?(x=w697) -> (x > 0?=w696:bool)
                    n273 = Not(x=w703) -> (.not. x?=w702:bool)
                    n274 = And(x=w701, y=w702) -> (x .and. y?=w700:bool)
                    n275 = Dequeue Element(queue=w706, timeout in ms (-1)=100, error in (no error)=w699) -> (element=w698:T8, error out=w692:errorcluster)  [unwired: 2 out]
                  }
                  frame #3 {
                    n276 = case shown="True" w719 {
                      tunnel: [w720 "FINALIZE"] -> w717
                      tunnel: w718 -> [w720 _]
                      frame False {
                      }
                      frame True {
                      }
                    }
                    n277 = local read "Number Of Channels"() -> (w715:i32)
                  }
                  frame #4 {
                    n278 = case shown="True" w735 {
                      tunnel: w736 -> [_ w773]
                      tunnel: w734 -> [_ w771]
                      tunnel: w733 -> [w739 w769]
                      tunnel: w732 -> [w738 w768]
                      tunnel: w731 -> [w740 w762]
                      tunnel: w730 -> [w741 w761]
                      tunnel: [w738 w756] -> w728
                      tunnel: [w741 w755] -> w727
                      tunnel: [w740 w754] -> w726
                      tunnel: [w739 w752] -> w725
                      tunnel: w723 -> [w737 _]
                      tunnel: [w737 w749] -> w722
                      frame False {
                      }
                      frame True {
                        n279 = Unbundle(w773) -> ("wfm info"=w749:T3, "wfm"=w772:i16[][], "Beam On?"=w747:bool, w746:i32)
                        n280 = flat-sequence {
                          tunnel: [w780] -> w770
                          tunnel: [w781] -> w766
                          tunnel: [w778] -> w748
                          tunnel: [w776] -> w745
                          tunnel: [w775] -> w744
                          tunnel: w746 -> [w776]
                          tunnel: w747 -> [w775]
                          tunnel: w768 -> [w774]
                          tunnel: w772 -> [w781]
                          tunnel: w749 -> [w779]
                          tunnel: w771 -> [_]
                          tunnel: [w774] -> w743
                          tunnel: w770 -> [w787]
                          tunnel: [w794] -> w767
                          tunnel: w766 -> [w794]
                          tunnel: [w793] -> w764
                          tunnel: [w792] -> w758
                          tunnel: w748 -> [w788]
                          tunnel: w745 -> [w784]
                          tunnel: w744 -> [w783]
                          tunnel: w743 -> [w782]
                          tunnel: [w782] -> w742
                          tunnel: w769 -> [w805]
                          tunnel: w767 -> [w804]
                          tunnel: [w803] -> w765
                          tunnel: w764 -> [w803]
                          tunnel: [w802] -> w763
                          tunnel: [w801] -> w759
                          tunnel: w758 -> [w801]
                          tunnel: [w800] -> w750
                          tunnel: w742 -> [w799]
                          tunnel: w765 -> [w817]
                          tunnel: w763 -> [w816]
                          tunnel: w762 -> [w815]
                          tunnel: [w814] -> w760
                          tunnel: w759 -> [w814]
                          tunnel: [w813] -> w757
                          tunnel: [w812] -> w753
                          tunnel: [w811] -> w751
                          tunnel: w750 -> [w811]
                          tunnel: w761 -> [w829]
                          tunnel: w760 -> [w828]
                          tunnel: w757 -> [w827]
                          tunnel: [w826] -> w756
                          tunnel: [w825] -> w755
                          tunnel: [w824] -> w754
                          tunnel: w753 -> [w824]
                          tunnel: [w823] -> w752
                          tunnel: w751 -> [w823]
                          frame #0 {
                            n281 = local read "number of resets"() -> (w780:i32)
                            n282 = Index Array(array=w779, index=0) -> (element=w778:T12)
                          }
                          frame #1 {
                            # "0. AbsoluteInitialX\n1. Xincrement\n2. Beam On? (1 yes, 0 no)\n3. Index of Maximum\n4. Rolling Transient Counter"
                            n283 = Boolean To (0,1)(Boolean=w783) -> (0, 1=w798:i16)
                            n284 = Unbundle(w788) -> ("actualSamples"=w792:i32, "absoluteInitialX"=w786:dbl, "xIncrement"=w785:dbl)  [unwired: 5 out]
                            n285 = To Double Precision Float(number=w784) -> (double precision float=w795:dbl)
                            n286 = To Double Precision Float(number=w787) -> (double precision float=w796:dbl)
                            n287 = Round To Nearest(number=w795) -> (nearest integer value=w789:dbl)
                            n288 = Round To Nearest(number=w796) -> (nearest integer value=w790:dbl)
                            n289 = To Double Precision Float(number=w798) -> (double precision float=w797:dbl)
                            n290 = Round To Nearest(number=w797) -> (nearest integer value=w791:dbl)
                            n291 = Build Array(w786, w785, w791, w789, w790) -> (w793:dbl[])
                          }
                          frame #2 {
                            n292 = Set File Position(refnum=w805, from (0:start)=enum16{"start", "end", "current"}."current", error in=w799) -> (refnum out=w809:refnum<file>, error out=w810:errorcluster)  [unwired: 1 in]
                            n293 = Write to Binary File(file (use dialog)=w809, data=w804, error in=w810, 5:FALSE ("prepend array or string size? (T)"), 9:T10."little-endian" ("byte order (0:big-endian, network order)")) -> (refnum out=w800:refnum<file>, error out=w802:errorcluster)  [unwired: 1 in, 1 out]
                          }
                          frame #3 {
                            n294 = Set File Position(refnum=w815, from (0:start)=enum16{"start", "end", "current"}."current", error in=w816) -> (refnum out=w821:refnum<file>, error out=w822:errorcluster)  [unwired: 1 in]
                            n295 = Write to Binary File(file (use dialog)=w821, data=w817, error in=w822, 5:FALSE ("prepend array or string size? (T)"), 9:T10."little-endian" ("byte order (0:big-endian, network order)")) -> (refnum out=w812:refnum<file>, error out=w813:errorcluster)  [unwired: 1 in, 1 out]
                          }
                          frame #4 {
                            n296 = Set File Position(refnum=w829, from (0:start)=enum16{"start", "end", "current"}."current", error in=w827) -> (refnum out=w833:refnum<file>, error out=w834:errorcluster)  [unwired: 1 in]
                            n297 = Write to Binary File(file (use dialog)=w833, data=w828, error in=w834, 5:FALSE ("prepend array or string size? (T)"), 9:T10."little-endian" ("byte order (0:big-endian, network order)")) -> (refnum out=w825:refnum<file>, error out=w826:errorcluster)  [unwired: 1 in, 1 out]
                          }
                        }
                      }
                    }
                  }
                  frame #5 {
                    n298 = Bundle("appended path"=w837, "refnum out"=w838, "refnum out"=w839, "refnum out"=w840) -> (w836:T4)  [unwired: 1 in]
                  }
                }
              }
              frame "FINALIZE" {
                n299 = flat-sequence {
                  tunnel: w863 -> [w885]
                  tunnel: w864 -> [w886]
                  tunnel: w865 -> [w887]
                  tunnel: w866 -> [w888]
                  tunnel: [w888] -> w851
                  tunnel: [w887] -> w850
                  tunnel: [w886] -> w849
                  tunnel: [w885] -> w848
                  tunnel: w847 -> [w873]
                  tunnel: w846 -> [w871]
                  tunnel: w845 -> [w869]
                  tunnel: [w868] -> w844
                  tunnel: [w867] -> w843
                  tunnel: w847 -> [_]
                  tunnel: [w890] -> w855
                  tunnel: [w898] -> w853
                  tunnel: w851 -> [w915]
                  tunnel: w850 -> [w914]
                  tunnel: w849 -> [w913]
                  tunnel: w848 -> [w912]
                  tunnel: w844 -> [w890]
                  tunnel: w843 -> [w889]
                  tunnel: w855 -> [w944]
                  tunnel: [w944] -> w854
                  tunnel: w853 -> [w940]
                  tunnel: [w930] -> w852
                  tunnel: w858 -> [w949]
                  tunnel: w854 -> [w947]
                  tunnel: [w946] -> w857
                  tunnel: w852 -> [w945]
                  tunnel: ["HOLDOFF"] -> w860
                  tunnel: w857 -> [w953]
                  tunnel: [w953] -> w856
                  frame #0 {
                    n300 = Unbundle(w873) -> ("name or relative path"=w872:string, w867:string)
                    n301 = Build Path(base path=w871, name or relative path=w872) -> (appended path=w870:path)
                    "RUN_FOLDER" <- w870
                    n302 = Build Path(base path=w870, name or relative path="RUN_TIMESTAMP_END.txt") -> (appended path=w879:path)
                    n303 = Get Date/Time In Seconds() -> (seconds since 1Jan1904=w883:timestamp)
                    n304 = Format Date/Time String(time format string (%c)="%H.%M.%S%8u", seconds (now)=w883) -> (date/time string=w884:string)  [unwired: 1 in]
                    n305 = Open/Create/Replace File(file path (use dialog)=w879, error in=w869, operation (0:open)=T9."open or create", access (0:read/write)=enum16{"read/write", "read-only", "write-only"}."read/write") -> (refnum out=w878:refnum<file>, error out=w881:errorcluster)  [unwired: 2 in, 1 out]
                    n306 = Write to Text File(file (use dialog)=w878, text=w884, error in=w881) -> (refnum out=w880:refnum<file>, error out=w882:errorcluster)  [unwired: 1 in, 1 out]
                    n307 = Close File(refnum=w880, error in=w882) -> (error out=w868:errorcluster)  [unwired: 1 out]
                  }
                  frame #1 {
                    n308 = local read "Channels Configured and Values"() -> (w903:string[][])
                    n309 = local read "Percent Threshold IND"() -> (w892:dbl)
                    n310 = local read "Sample Rate IND"() -> (w897:dbl)
                    n311 = local read "AUTOMITIGATION ENABLED IND"() -> (w909:bool)
                    n312 = local read "Present Mitigation Information"() -> (w908:string)
                    n313 = local read "Nominal Current IND"() -> (w894:dbl)
                    n314 = Reciprocal(x=w897) -> (1/x=w906:dbl)
                    n315 = Delete From Array(array=w903, index (row)=0) -> (array with subset deleted=w901:string[][])  [unwired: 2 in, 1 out]
                    n316 = Multiply(x=w892, y=100.0) -> (x*y=w891:dbl)
                    n317 = local read "channels IND"() -> (w896:string)
                    n318 = local read "wfm info IND"() -> (w895:T3)
                    n319 = Bundle("AUTOMITIGATION ENABLED IND"=w909, "Present Mitigation Information"=w908) -> (w907:T13)  [unwired: 1 in]
                    n320 = Number To Fractional String(number=w894) -> (F-format string=w904:string)  [unwired: 3 in]
                    n321 = Number To Fractional String(number=w906) -> (F-format string=w905:string)  [unwired: 3 in]
                    n322 = Number To Fractional String(number=w897) -> (F-format string=w910:string)  [unwired: 3 in]
                    n323 = Number To Fractional String(number=w891) -> (F-format string=w911:string)  [unwired: 3 in]
                    n324 = Index Array(array=w901, index (col)=1 ("disabled index (col)")) -> (element=w899:string[])  [unwired: 1 in]
                    n325 = disable-structure shown="Enabled" {
                      disable-tunnel: w915 -> [w928]
                      disable-tunnel: w914 -> [w927]
                      disable-tunnel: w913 -> [w923]
                      disable-tunnel: w912 -> [w922]
                      disable-tunnel: w911 -> [w918]
                      disable-tunnel: w910 -> [w919]
                      disable-tunnel: w907 -> [w916]
                      disable-tunnel: w905 -> [w920]
                      disable-tunnel: w904 -> [w921]
                      disable-tunnel: w899 -> [w929]
                      disable-tunnel: [w925] -> w898
                      disable-tunnel: w896 -> [w926]
                      disable-tunnel: w895 -> [w917]
                      disable-tunnel: w889 -> [w924]
                      frame Enabled {
                        n326 = call "StandAloneTransient_TestBenchParametersArrayCreation.vi"("Input Voltage Array"=w929, "Board Number"=w924, "DUT"=w923, "Nominal Current (A)"=w922, "XINC"=w921, "Test Type"=w920, "Effective LET"=w928, "Sample Rate (SPS)"=w919, "Threshold Percentage (%)"=w918, "Ion (ex. Kr)"=w927, "wfm info single capture"=w917, "Channel"=w926, "Mitigation Information"=w916) -> ("Array"=w925:string[][])  [unwired: 6 in]
                      }
                    }
                  }
                  frame #2 {
                    n327 = local read "Channel To Mitigate (0-7) IND"() -> (w939:i32)
                    n328 = Add(x=2, y=w939) -> (x+y=w937:i32)
                    n329 = local read "number of resets"() -> (w934:i32)
                    n330 = Index Array(array=w940, index (row)=w937, index (col)=0 ("disabled index (col)")) -> (element=w936:string)
                    n331 = Build Array("Channel_to_mitigate", w936) -> (w942:string[])
                    n332 = Number To Decimal String(number=w934) -> (decimal integer string=w933:string)  [unwired: 1 in]
                    n333 = Insert Into Array(array=w940, new element=w942) -> (w935:string[][])  [unwired: 2 in]
                    n334 = Build Array("Number_of_resets" ("element"), w933) -> (w931:string[])
                    n335 = Insert Into Array(array=w935, new element=w931) -> (w930:string[][])  [unwired: 2 in]
                  }
                  frame #3 {
                    n336 = call-poly <vilib>:"Write Delimited Spreadsheet.vi"("file path (dialog if empty)"=w949, "format (%s)"="%s" ("format (%.3f)"), "2D data"=w945, "append to file? (new file:F)"=FALSE, "error in (no error)"=w947, "transpose? (no:F)"=FALSE, "delimiter (\\t)"="," ("delimiter (\\t)")) -> ("error out"=w946:errorcluster)  [unwired: 7 in, 1 out]
                  }
                  frame #4 {
                  }
                }
              }
              frame "HOLDOFF", Default {
                n337 = Equal?(x=w956, y=0) -> (x = y?=w957:bool)
                n338 = local read "INITIALIZED"() -> (w968:bool)
                n339 = Or(x=w957, y="APPLYPATH") -> (x .or. y?=w958:bool)
                n340 = case shown="False" w968 {
                  tunnel: w958 -> [w974 _]
                  tunnel: w970 -> [w973 w978]
                  tunnel: [w972 w978] -> w969
                  tunnel: [w971 "FOLDERCREATION"] -> w967
                  tunnel: w966 -> [w971 _]
                  frame False {
                    n341 = case shown="True" w974 {
                      tunnel: w973 -> [w975 _]
                      tunnel: [w975 "INPUTPATH"] -> w972
                      frame False {
                      }
                      frame True {
                      }
                    }
                  }
                  frame True {
                  }
                }
              }
            }
            "CURRENTPATH" <- w460
            n342 = local read "FINISH PROGRAM"() -> (w462:bool)
          }
          n343 = while {
            shift-right: [w2142] -> _
            shift-left: "STANDBY" -> [w2144]
            shift-right: [w2140] -> _
            shift-left: FALSE -> [w2141]
            tunnel: "PSU" -> [w2138]
            shift-right: [w2139] -> w416
            shift-left: w394 -> [w2137]
            shift-right: [w2125] -> _
            shift-left: string[][] [["Unconfirmed"]] -> [w2124]
            shift-right: [w2123] -> _
            shift-left: "Unconfirmed" ("read buffer") -> [w2122]
            tunnel: "resource name" -> [w2119]
            shift-right: [w2113] -> _
            shift-left: FALSE -> [w2112]
            i -> [w2109]
            stop <- "stop" stop-if-true
            # "Implement this in the enable state eventually to apply functional resetting of the device"
            n344 = Greater?(x=w2109, y=2000000000) -> (0:→"RESTART PROGRAM SOON (DATACOLLECT)":bool)
            n345 = Equal?(x=0, y=w2109) -> (x = y?=w2115:bool)
            n346 = Or(x="APPLY POWER SETTINGS", y=w2115) -> (x .or. y?=w2117:bool)
            n347 = Build Array("Voltage Channel 1", "Voltage Channel 2", "Voltage Channel 3") -> (w2130:dbl[])
            n348 = Build Array("Current Limit Channel 1", "Current Limit Channel 2", "Current Limit Channel 3") -> (w2126:dbl[])
            n349 = case shown="\"STANDBY\", Default" w2144 {
              tunnel: ["STANDBY" w2291 "STANDBY" "STANDBY" "STANDBY" "STANDBY"] -> w2142
              tunnel: w2141 -> [w2253 w2285 w2371 w2385 w2396 w2405]
              tunnel: [w2252 w2288 w2371 w2385 w2396 w2405] -> w2140
              tunnel: w2137 -> [w2263 w2286 w2368 w2377 w2389 w2398]
              tunnel: [w2262 w2287 w2366 w2376 w2386 w2397] -> w2139
              tunnel: w2138 -> [w2260 _ w2369 _ w2387 _]
              tunnel: "POWER ON" -> [_ w2281 _ _ _ _]
              tunnel: w2117 -> [_ w2284 _ _ _ _]
              tunnel: "Combination" -> [w2251 _ _ _ _ _]
              tunnel: "Channels to Parallelize (if selected)" -> [w2250 _ _ _ _ _]
              tunnel: w2130 -> [w2249 _ _ _ _ _]
              tunnel: w2126 -> [w2248 _ _ _ _ _]
              tunnel: [w2247 w2283 w2364 w2384 w2394 w2404] -> w2125
              tunnel: w2124 -> [_ w2283 w2364 w2384 w2394 w2404]
              tunnel: [w2246 w2282 w2367 w2383 w2393 w2403] -> w2123
              tunnel: w2122 -> [_ w2282 w2367 w2383 w2393 w2403]
              tunnel: w2119 -> [_ _ _ w2380 w2391 w2400]
              tunnel: "NIDCPOWER_CHAN" -> [_ _ _ w2379 w2390 w2399]
              tunnel: "NIDCPOWER_VOLT" -> [_ _ _ w2378 _ _]
              tunnel: "DC Power On" -> [_ w2280 _ _ _ _]
              tunnel: [w2245 w2279 w2365 TRUE FALSE FALSE] -> w2113
              tunnel: w2112 -> [w2245 w2278 w2365 _ _ _]
              frame "POWER_APPLY" {
                # "Creating the Voltage/Current Array that is passed into the keithley 2230 block"
                n350 = Build Array(w2249, w2248) -> (w2265:dbl[][])
                n351 = Transpose 2D Array(2D array=w2265) -> (transposed array=w2264:dbl[][])
                n352 = disable-structure shown="Enabled" {
                  disable-tunnel: w2264 -> [w2268]
                  disable-tunnel: w2263 -> [w2271]
                  disable-tunnel: [w2272] -> w2262
                  disable-tunnel: [w2275] -> w2261
                  disable-tunnel: w2260 -> [w2267]
                  disable-tunnel: [w2274] -> w2259
                  disable-tunnel: w2253 -> [w2277]
                  disable-tunnel: [w2276] -> w2252
                  disable-tunnel: w2251 -> [w2269]
                  disable-tunnel: w2250 -> [w2270]
                  disable-tunnel: [w2273] -> w2246
                  frame Enabled {
                    n353 = call "StandAloneTransient_Dynamic_Keithley2230_PSU_Configuration_V1.vi"("VISA resource name"=w2267, "POWER STATUS IN"=w2277, "Input Array (Voltage,Current_Limit)"=w2268, "Combination Scheme"=w2269, "Which Channels to Parallelize"=w2270, "error in"=w2271) -> ("POWER STATUS OUT"=w2276:bool, "Array 4"=w2275:dbl[][], "Array"=w2274:string[], "read buffer"=w2273:string, "error out"=w2272:errorcluster)  [unwired: 5 in]
                  }
                }
                n354 = Number To Fractional String(number=w2261) -> (F-format string=w2257:string[][])  [unwired: 3 in]
                n355 = Insert Into Array(array=w2257, index (col)=0 ("disabled index (col)"), new element=w2259) -> (w2254:string[][])  [unwired: 1 in]
                n356 = Insert Into Array(array=w2254, index (row)=0, new element=string[] ["CHANNEL", "VOLTAGE", "CURRENT LIMIT"] ("new element/subarray")) -> (w2247:string[][])  [unwired: 1 in]
              }
              frame "STANDBY", Default {
                n357 = Not(x=w2285) -> (.not. x?=w2289:bool)
                n358 = And(x=w2289, y=w2281) -> (x .and. y?=w2290:bool)
                n359 = case shown="False" w2290 {
                  selector: w2290 -> [_ w2363]
                  tunnel: [w2306 "POWER_ON"] -> w2291
                  tunnel: [w2301 w2363] -> w2288
                  tunnel: [w2305 w2361] -> w2287
                  tunnel: w2286 -> [w2304 w2361]
                  tunnel: w2285 -> [w2303 _]
                  tunnel: w2281 -> [w2302 _]
                  tunnel: w2284 -> [w2300 _]
                  tunnel: w2281 -> [w2299 _]
                  tunnel: w2280 -> [w2298 _]
                  tunnel: [w2292 w2360] -> w2279
                  tunnel: w2278 -> [w2295 w2360]
                  tunnel: w2278 -> [w2293 _]
                  frame False {
                    n360 = And(x=w2298, y=w2299) -> (x .and. y?=w2297:bool)
                    n361 = Not(x=w2295) -> (.not. x?=w2294:bool)
                    n362 = And(x=w2297, y=w2294) -> (x .and. y?=w2296:bool)
                    n363 = case shown="False" w2296 {
                      selector: w2296 -> [w2313 _]
                      tunnel: [w2320 "ENABLE_ON"] -> w2306
                      tunnel: [w2319 w2357] -> w2305
                      tunnel: w2304 -> [w2318 w2357]
                      tunnel: w2303 -> [w2317 w2358]
                      tunnel: w2302 -> [w2316 _]
                      tunnel: [w2315 w2358] -> w2301
                      tunnel: w2300 -> [w2314 _]
                      tunnel: w2298 -> [w2310 _]
                      tunnel: w2295 -> [w2311 _]
                      tunnel: w2293 -> [w2308 w2356]
                      tunnel: [w2312 w2356] -> w2292
                      frame False {
                        n364 = Not And(1:w2310, 2:w2311) -> (0:w2309:bool)
                        n365 = And(x=w2309, y=w2308) -> (x .and. y?=w2307:bool)
                        n366 = case shown="False" w2307 {
                          tunnel: [w2329 "ENABLE_OFF"] -> w2320
                          tunnel: [w2328 w2353] -> w2319
                          tunnel: w2318 -> [w2327 w2353]
                          tunnel: w2317 -> [w2326 w2355]
                          tunnel: w2316 -> [w2325 _]
                          tunnel: [w2324 w2355] -> w2315
                          tunnel: w2314 -> [w2323 _]
                          tunnel: w2313 -> [_ _]
                          tunnel: [w2322 FALSE] -> w2312
                          tunnel: w2308 -> [w2321 _]
                          frame False {
                            n367 = case shown="False" w2323 {
                              tunnel: [w2339 "POWER_APPLY"] -> w2329
                              tunnel: [w2338 w2350] -> w2328
                              tunnel: w2327 -> [w2337 w2350]
                              tunnel: w2326 -> [w2332 w2349]
                              tunnel: w2325 -> [w2334 _]
                              tunnel: [w2333 w2349] -> w2324
                              tunnel: [w2331 w2348] -> w2322
                              tunnel: w2321 -> [w2330 w2348]
                              frame False {
                                n368 = Not(x=w2334) -> (.not. x?=w2336:bool)
                                n369 = And(x=w2336, y=w2332) -> (x .and. y?=w2335:bool)
                                n370 = case shown="False" w2335 {
                                tunnel: ["STANDBY" "POWER_OFF"] -> w2339
                                tunnel: [w2342 w2347] -> w2338
                                tunnel: w2337 -> [w2342 w2347]
                                tunnel: [w2341 FALSE] -> w2333
                                tunnel: w2332 -> [w2341 _]
                                tunnel: [w2340 FALSE] -> w2331
                                tunnel: w2330 -> [w2340 _]
                                frame False {
                                }
                                frame True {
                                }
                                }
                              }
                              frame True {
                              }
                            }
                          }
                          frame True {
                          }
                        }
                      }
                      frame True {
                      }
                    }
                  }
                  frame True {
                  }
                }
              }
              frame "POWER_ON" {
                n371 = disable-structure shown="Enabled" {
                  disable-tunnel: w2369 -> [w2374]
                  disable-tunnel: w2368 -> [w2373]
                  disable-tunnel: [w2372] -> w2366
                  frame Enabled {
                    n372 = call "StandAloneTransient_Keithley2230_PSU_POWER_ON_V1.vi"("error in (no error)"=w2373, "VISA resource name"=w2374) -> ("error out"=w2372:errorcluster)  [unwired: 9 in]
                  }
                }
              }
              frame "ENABLE_ON" {
                n373 = call "StandAloneTransient_NIDCPOWER_PSU_POWER_ON_V1.vi"("error in"=w2377, "voltage level"=w2378, "channel name"=w2379, "resource name"=w2380) -> ("error out"=w2376:errorcluster, "current limit"=→"current limit ind":dbl)  [unwired: 6 in]
              }
              frame "POWER_OFF" {
                n374 = call "StandAloneTransient_NIDCPOWER_PSU_POWER_OFF_V1.vi"("error in"=w2389, "channel name"=w2390, "resource name"=w2391) -> ("eRROR OUT"=w2388:errorcluster)  [unwired: 8 in]
                n375 = call "StandAloneTransient_Keithley2230_PSU_POWER_OFF_V1.vi"("error in (no error)"=w2388, "VISA resource name"=w2387) -> ("error out"=w2386:errorcluster)  [unwired: 9 in]
              }
              frame "ENABLE_OFF" {
                n376 = call "StandAloneTransient_NIDCPOWER_PSU_POWER_OFF_V1.vi"("error in"=w2398, "channel name"=w2399, "resource name"=w2400) -> ("eRROR OUT"=w2397:errorcluster)  [unwired: 8 in]
              }
            }
            "POWER STATE" <- w2140
            "Channels Configured and Values" <- w2125
            "Present Channel Configuration" <- w2123
            "ENABLE STATE" <- w2113
            n377 = disable-structure shown="Disabled" {
              disable-tunnel: _ -> [w2150 _]
              disable-tunnel: _ -> [w2148 _]
              disable-tunnel: _ -> [w2146 _]
              disable-tunnel: [w2145 _] -> _
              frame Disabled {
                # "DC Power Resource"
                # "VISA PSU"
                # "Overthreshold counter"
                n378 = while {
                  tunnel: w2150 -> [w2167]
                  shift-right: [w2169] -> w2145
                  shift-left: w2146 -> [w2168]
                  tunnel: [w2167] -> _
                  shift-right: [w2165] -> _
                  shift-left: "NONE" -> [w2166]
                  tunnel: w2148 -> [w2164]
                  shift-right: [w2151] -> _
                  shift-left: 0 -> [w2155]
                  stop <- w2170 stop-if-true
                  # "ADD THE AUTOMITIGATION PARAMETERS WITHIN THE TEST BENCH"
                  n379 = local read "Collecting Data"() -> (w2153:bool)
                  n380 = local read "EXCEED DURATION"() -> (w2158:bool)
                  n381 = local read "FOLDERCREATED"() -> (w2152:bool)
                  n382 = And(x="AUTOMITIGATION ENABLED", y=w2153) -> (x .and. y?=w2156:bool)
                  n383 = And(x=w2156, y=w2158) -> (x .and. y?=w2159:bool)
                  n384 = case shown="True" w2152 {
                    tunnel: [w2171 0] -> w2154
                    tunnel: w2155 -> [w2171 _]
                    frame False {
                    }
                    frame True {
                    }
                  }
                  n385 = Or(x="FORCED RESET", y=w2159) -> (x .or. y?=w2160:bool)
                  n386 = case shown="False" "CHANGE MITIGATION" {
                    tunnel: w2160 -> [w2181 _]
                    tunnel: [w2175 w2239] -> w2169
                    tunnel: w2168 -> [w2180 w2239]
                    tunnel: w2166 -> [w2179 _]
                    tunnel: w2167 -> [w2178 _]
                    tunnel: [w2177 w2240] -> w2165
                    tunnel: w2164 -> [w2176 _]
                    tunnel: "Mitigation" -> [_ w2238]
                    tunnel: w2154 -> [w2174 w2237]
                    tunnel: [w2173 w2237] -> w2151
                    frame False {
                      n387 = case shown="True" w2181 {
                        tunnel: w2178 -> [_ w2194]
                        tunnel: [w2184 w2193] -> w2175
                        tunnel: w2180 -> [w2184 w2192]
                        tunnel: w2179 -> [w2183 w2191]
                        tunnel: [w2183 w2190] -> w2177
                        tunnel: w2176 -> [_ w2189]
                        tunnel: [w2182 w2185] -> w2173
                        tunnel: w2174 -> [w2182 w2186]
                        frame False {
                        }
                        frame True {
                          n388 = local read "NIDCPOWER_CHAN_CONF"() -> (w2188:string)
                          n389 = local read "NIDCPOWER_VOLT_CONF"() -> (w2187:dbl)
                          n390 = case shown="\"Hardware\"" w2191 {
                            selector: w2191 -> [w2206 w2218 w2221 w2230]
                            tunnel: w2194 -> [w2203 w2215 _ _]
                            tunnel: [w2195 w2207 w2220 w2227] -> w2193
                            tunnel: w2192 -> [w2201 w2213 w2220 w2228]
                            tunnel: [w2206 w2218 w2221 w2230] -> w2190
                            tunnel: w2189 -> [w2199 w2211 _ w2229]
                            tunnel: w2188 -> [w2198 w2210 _ w2225]
                            tunnel: w2187 -> [w2197 w2209 _ w2224]
                            tunnel: [w2204 w2216 w2219 w2222] -> w2185
                            tunnel: w2186 -> [w2205 w2217 w2219 w2223]
                            frame "PowerCycle" {
                              n391 = call "StandAloneTransient_NIDCPOWER_PSU_POWER_OFF_V1.vi"("error in"=w2201, "channel name"=w2198, "resource name"=w2199) -> ("eRROR OUT"=w2200:errorcluster)  [unwired: 8 in]
                              n392 = Increment(x=w2205) -> (x+1=w2204:i32)
                              n393 = call "StandAloneTransient_Keithley2230_PSU_POWER_CYCLE_V1.vi"("error in (no error)"=w2200, "milliseconds to wait"=u32 200, "VISA Refnum in"=w2203) -> ("error out"=w2196:errorcluster)  [unwired: 8 in]
                              n394 = call "StandAloneTransient_NIDCPOWER_PSU_POWER_ON_V1.vi"("error in"=w2196, "voltage level"=w2197, "channel name"=w2198, "resource name"=w2199) -> ("error out"=w2195:errorcluster)  [unwired: 6 in, 1 out]
                            }
                            frame "Hardware" {
                              n395 = call "StandAloneTransient_NIDCPOWER_PSU_POWER_OFF_V1.vi"("error in"=w2213, "channel name"=w2210, "resource name"=w2211) -> ("eRROR OUT"=w2212:errorcluster)  [unwired: 8 in]
                              n396 = Increment(x=w2217) -> (x+1=w2216:i32)
                              n397 = call "StandAloneTransient_Keithley2230_PSU_POWER_CYCLE_V1.vi"("error in (no error)"=w2212, "milliseconds to wait"=u32 200, "VISA Refnum in"=w2215) -> ("error out"=w2208:errorcluster)  [unwired: 8 in]
                              n398 = call "StandAloneTransient_NIDCPOWER_PSU_POWER_ON_V1.vi"("error in"=w2208, "voltage level"=w2209, "channel name"=w2210, "resource name"=w2211) -> ("error out"=w2207:errorcluster)  [unwired: 6 in, 1 out]
                            }
                            frame "NONE", Default {
                            }
                            frame "EnableCircuit" {
                              n399 = disable-structure shown="Enabled" {
                                disable-tunnel: w2229 -> [w2235]
                                disable-tunnel: w2228 -> [w2232]
                                disable-tunnel: [w2231] -> w2227
                                disable-tunnel: u32 200 ("milliseconds to wait") -> [w2233]
                                disable-tunnel: w2225 -> [w2234]
                                disable-tunnel: w2224 -> [w2236]
                                frame Enabled {
                                n400 = call "StandAloneTransient_NIDCPOWER_PSU_POWER_CYCLE_V1.vi"("NIDCPOWER_VOLT_CONF"=w2236, "error in (no error)"=w2232, "milliseconds to wait"=w2233, "NIDCPOWER_CHAN_CONF"=w2234, "IVI Refnum in"=w2235) -> ("error out"=w2231:errorcluster)  [unwired: 6 in]
                                }
                              }
                              n401 = Increment(x=w2223) -> (x+1=w2222:i32)
                            }
                          }
                        }
                      }
                    }
                    frame True {
                      n402 = case shown="3" w2238 {
                        tunnel: ["NONE" "HARDWARE" "EnableCircuit" "PowerCycle"] -> w2240
                        frame 0, Default {
                        }
                        frame 1 {
                        }
                        frame 3 {
                        }
                        frame 2 {
                        }
                      }
                    }
                  }
                  "Present Mitigation Information" <- w2165
                  "number of resets" <- w2151
                  n403 = local read "FINISH PROGRAM"() -> (w2170:bool)
                  "AUTOMITIGATION ENABLED IND" <- "AUTOMITIGATION ENABLED"
                }
              }
              frame Enabled {
              }
            }
            "FINISH PROGRAM" <- "stop"
            "NIDCPOWER_CHAN_CONF" <- "NIDCPOWER_CHAN"
            "NIDCPOWER_VOLT_CONF" <- "NIDCPOWER_VOLT"
          }
          n404 = while {
            shift-right: [w1020] -> _
            shift-left: "HOLDBY" -> [w1021]
            shift-right: [w1018] -> w414
            shift-left: w394 -> [w1016]
            tunnel: w418 -> [w1017]
            tunnel: [w1019] -> w419
            tunnel: w398 -> [w1011]
            shift-right: [w995] -> _
            shift-left: 0 ("index") -> [w992]
            shift-right: [w997] -> _
            shift-left: 0.0 ("Nominal Current") -> [w993]
            shift-right: [w996] -> _
            shift-left: 0 ("index") -> [w994]
            shift-right: [w998] -> _
            shift-left: FALSE ("x > y?") -> [w991]
            shift-right: [w990] -> _
            shift-left: 0 -> [w989]
            shift-right: [w988] -> _
            shift-left: T7 {"array"=[], "array"=[], "array"=[], "array"=[], "array"=[], "array"=[], "array"=[], "array"=[]} -> [w987]
            shift-right: [w984] -> _
            shift-left: 3000 ("y") -> [w986]
            shift-right: [w982] -> _
            shift-left: "" -> [w981]
            i -> [w980]
            stop <- w1022 stop-if-true
            n405 = Divide(x="TRANSIENT TIME DURATION (ms)", y=1000.0) -> (x/y=w999:dbl)
            n406 = Divide(x="Percent Threshold", y=100.0) -> (x/y=w1000:dbl)
            n407 = Greater?(x=w980, y=2000000000) -> (0:→"RESTART PROGRAM SOON (DATASTORE)":bool)
            n408 = case shown="\"COLLECTION16\"" w1021 {
              selector: w1021 -> [_ _ w1340 w1496 _]
              tunnel: [w1047 w1199 w1339 w1498 w2103] -> w1020
              tunnel: [w1053 w1196 w1344 w1499 w2102] -> w1019
              tunnel: [w1052 w1195 w1341 w1500 w2101] -> w1018
              tunnel: w1017 -> [w1051 w1204 w1343 w1502 w2102]
              tunnel: w1016 -> [w1050 w1203 w1342 w1501 w2101]
              tunnel: "BEGIN RECORDING" -> [_ _ _ w1497 w2100]
              tunnel: "channels" -> [w1046 w1188 w1330 w1495 _]
              tunnel: "Min. Sample Rate" -> [w1041 w1202 _ _ _]
              tunnel: "Vertical Range (V)" -> [w1049 w1201 _ _ _]
              tunnel: "Max Points per Fetch" -> [_ _ _ w1494 _]
              tunnel: w1011 -> [_ _ _ w1493 _]
              tunnel: "INTIALIZE SCOPE" -> [_ _ _ _ w2099]
              tunnel: "50 ohm vertical range (V)" -> [w1045 w1197 _ _ _]
              tunnel: "Channel 0 50 ohms?" -> [w1044 w1198 _ _ _]
              tunnel: "min record length" -> [w1042 w1194 _ _ _]
              tunnel: "vertical coupling" -> [w1043 w1193 _ _ _]
              tunnel: w994 -> [_ w1190 w1334 w1492 w2097]
              tunnel: "Nominal Mitigation Value" -> [_ _ _ w1491 _]
              tunnel: w1000 -> [_ _ _ w1490 _]
              tunnel: w999 -> [_ _ _ w1489 _]
              tunnel: w992 -> [_ w1189 w1335 w1488 w2095]
              tunnel: w993 -> [_ w1191 w1336 w1487 w2096]
              tunnel: w991 -> [_ w1192 w1337 w1486 w2098]
              tunnel: [FALSE ("x > y?") w1192 w1337 w1485 w2098] -> w998
              tunnel: [0.0 ("Nominal Current") w1191 w1336 w1484 w2096] -> w997
              tunnel: [0 ("index") w1190 w1334 w1483 w2097] -> w996
              tunnel: [0 ("index") w1189 w1335 w1482 w2095] -> w995
              tunnel: [w1036 w1187 w1329 w1481 w2094] -> w990
              tunnel: w989 -> [_ _ w1329 w1481 w2094]
              tunnel: [T7 {"array"=[], "array"=[], "array"=[], "array"=[], "array"=[], "array"=[], "array"=[], "array"=[]} w1186 w1333 w1480 w2093] -> w988
              tunnel: w987 -> [_ w1186 w1333 w1479 w2093]
              tunnel: w980 -> [_ _ _ w1478 _]
              tunnel: w986 -> [_ w1185 w1332 w1477 w2092]
              tunnel: "Min. Sample Rate" -> [w1034 _ _ _ _]
              tunnel: [w1031 w1185 w1332 w1477 w2092] -> w984
              tunnel: [w1023 w1170 w1331 w1476 w2091] -> w982
              tunnel: w981 -> [_ _ w1331 w1475 w2091]
              frame "INITIALIZE" {
                n409 = flat-sequence {
                  tunnel: w1041 -> [w1060]
                  tunnel: w1043 -> [w1061]
                  tunnel: w1044 -> [w1062]
                  tunnel: w1046 -> [w1057]
                  tunnel: w1049 -> [w1063]
                  tunnel: w1050 -> [w1055]
                  tunnel: w1051 -> [w1064]
                  tunnel: [w1064] -> w1030
                  tunnel: [w1054] -> w1029
                  tunnel: [w1063] -> w1028
                  tunnel: [w1056] -> w1027
                  tunnel: [w1062] -> w1026
                  tunnel: [w1061] -> w1025
                  tunnel: [w1060] -> w1024
                  tunnel: [w1149] -> w1053
                  tunnel: [w1148] -> w1052
                  tunnel: ["WAIT4FOLDER"] -> w1048
                  tunnel: w1045 -> [w1131]
                  tunnel: w1042 -> [w1124]
                  tunnel: [w1122] -> w1036
                  tunnel: w1030 -> [w1147]
                  tunnel: w1029 -> [w1146]
                  tunnel: w1028 -> [w1145]
                  tunnel: w1027 -> [w1121]
                  tunnel: w1026 -> [w1130]
                  tunnel: w1025 -> [w1129]
                  tunnel: w1024 -> [w1123]
                  tunnel: [w1121] -> w1023
                  frame #0 {
                    n410 = while {
                      shift-right: [w1080] -> _
                      shift-left: w1057 -> [w1081]
                      shift-right: [w1066] -> _
                      shift-left: 0 -> [w1072]
                      shift-right: [w1074] -> w1056
                      shift-left: "" -> [w1070]
                      tunnel: [w1080] -> _ mode=indexing
                      tunnel: w1055 -> [w1069]
                      tunnel: [w1068] -> w1054
                      i -> [w1079]
                      stop <- w1078 stop-if-true
                      n411 = flat-sequence {
                        tunnel: w1081 -> [w1091]
                        tunnel: w1079 -> [_]
                        tunnel: [w1089] -> w1077
                        tunnel: [w1082] -> w1076
                        tunnel: [w1083] -> w1075
                        tunnel: [w1088] -> w1073
                        tunnel: w1072 -> [w1088]
                        tunnel: [w1087] -> w1071
                        tunnel: w1070 -> [w1087]
                        tunnel: [w1082] -> w1065
                        tunnel: w1077 -> [w1103]
                        tunnel: w1076 -> [w1094]
                        tunnel: w1075 -> [w1102]
                        tunnel: w1073 -> [w1100]
                        tunnel: w1071 -> [w1099]
                        tunnel: w1069 -> [w1098]
                        tunnel: [w1103] -> w1080
                        tunnel: [w1094] -> w1078
                        tunnel: [w1101] -> w1074
                        tunnel: [w1097] -> w1068
                        tunnel: [w1096] -> w1067
                        tunnel: w1065 -> [w1095]
                        frame #0 {
                          n412 = Match Pattern(string=w1091, regular expression=",") -> (before substring=w1086:string, after substring=w1089:string, offset past match=w1093:i32)  [unwired: 1 in, 1 out]
                          n413 = Equal?(x=w1086, y="") -> (x = y?=w1084:bool)
                          n414 = Equal?(x=w1093, y=-1) -> (x = y?=w1082:bool)
                          n415 = And(x=w1082, y=w1084) -> (x .and. y?=w1083:bool)
                        }
                        frame #1 {
                          n416 = case shown="False" w1102 {
                            tunnel: [w1104 ""] -> w1101
                            tunnel: w1100 -> [w1109 w1118]
                            tunnel: w1099 -> [w1107 _]
                            tunnel: [w1109 w1118] -> w1096
                            tunnel: w1098 -> [w1108 _]
                            tunnel: [w1108 errorcluster {"status"=TRUE, "code"=-5, "source"="No Channel Parameter: Ensure you have entered channel names in on \"channels (comma separated)\" AND there is no comma at the end of the string in \"channels (comma separated)"} ("error out")] -> w1097
                            tunnel: w1095 -> [_ _]
                            tunnel: w1094 -> [w1105 _]
                            frame False {
                              n417 = Number To Decimal String(number=w1109) -> (decimal integer string=w1106:string)  [unwired: 1 in]
                              n418 = case shown="True" w1105 {
                                tunnel: w1107 -> [w1113 w1116]
                                tunnel: w1106 -> [w1112 w1115]
                                tunnel: [w1110 w1114] -> w1104
                                frame False {
                                n419 = Concatenate Strings(w1113, w1112, "," ("string")) -> (w1110:string)
                                }
                                frame True {
                                n420 = Concatenate Strings(w1116, w1115) -> (w1114:string)
                                }
                              }
                            }
                            frame True {
                            }
                          }
                        }
                      }
                      n421 = Increment(x=w1067) -> (x+1=w1066:i32)
                    }
                  }
                  frame #1 {
                    w1150 = u32 0 items=["1 mega ohm"=0, "50 ohms"=2] ("input impedance")
                    w1155 = 388 items=["Start"=482, "Trigger"=483, "Pretrigger"=477, "Now"=481, "Read Pointer"=388] ("Fetch:Fetch Relative To")
                    # "3"
                    n422 = String Length(string=w1121) -> (length=w1143:i32)
                    n423 = Match Pattern(string=w1121, regular expression="0") -> (offset past match=w1133:i32)  [unwired: 1 in, 3 out]
                    n424 = call <instrlib>:"niScope Configure Vertical.vi"("instrument handle"=w1147, "vertical coupling"=w1129, "channels"=w1121, "vertical range"=w1145, "error in"=w1146) -> ("instrument handle out"=w1152:refnum<k15>, "error out"=w1151:errorcluster)  [unwired: 9 in]
                    n425 = Quotient & Remainder(x=w1143, y=2) -> (x-y*floor(x/y)=w1140:i32, floor(x/y)=w1141:i32)
                    n426 = Not Equal?(x=w1133, y=-1) -> (x != y?=w1134:bool)
                    n427 = And(x=w1130, y=w1134) -> (x .and. y?=w1135:bool)
                    n428 = Add(x=w1140, y=w1141) -> (x+y=w1122:i32)
                    n429 = call <instrlib>:"niScope Configure Chan Characteristics.vi"("instrument handle"=w1152, "channels"=w1121, "input impedance"=w1150, "maximum input frequency"=0.0, "error in"=w1151) -> ("instrument handle out"=w1138:refnum<k15>, "error out"=w1137:errorcluster)  [unwired: 9 in]
                    n430 = case shown="True" w1135 {
                      tunnel: [w1159 w1169] -> w1128
                      tunnel: [w1158 w1168] -> w1127
                      tunnel: w1138 -> [w1159 w1163]
                      tunnel: w1137 -> [w1158 w1162]
                      tunnel: w1131 -> [_ w1160]
                      frame False {
                      }
                      frame True {
                        w1166 = u32 2 items=["1 mega ohm"=0, "50 ohms"=2] ("input impedance")
                        w1161 = "0" ("channels")
                        n431 = call <instrlib>:"niScope Configure Vertical.vi"("instrument handle"=w1163, "channels"=w1161, "vertical range"=w1160, "error in"=w1162) -> ("instrument handle out"=w1165:refnum<k15>, "error out"=w1164:errorcluster)  [unwired: 10 in]
                        n432 = call <instrlib>:"niScope Configure Chan Characteristics.vi"("instrument handle"=w1165, "channels"=w1161, "input impedance"=w1166, "maximum input frequency"=0.0, "error in"=w1164) -> ("instrument handle out"=w1169:refnum<k15>, "error out"=w1168:errorcluster)  [unwired: 9 in]
                      }
                    }
                    n433 = call <instrlib>:"niScope Configure Horizontal Timing.vi"("instrument handle"=w1128, "min sample rate"=w1123, "error in"=w1127, "min record length"=w1124) -> ("instrument handle out"=w1125:refnum<k15>, "error out"=w1126:errorcluster)  [unwired: 10 in]
                    n434 = call-poly <instrlib>:"niScope Configure Trigger (poly).vi"("instrument handle"=w1125, "error in"=w1126) -> ("instrument handle out"=w1154:refnum<k15>, "error out"=w1153:errorcluster)  [unwired: 12 in]
                    n435 = call <instrlib>:"niScope Initiate Acquisition.vi"("instrument handle"=w1154, "error in"=w1153) -> ("instrument handle out"=w1156:refnum<k15>, "error out"=w1157:errorcluster)  [unwired: 12 in]
                    n436 = property class="niScope" props=["Fetch:Fetch Relative To", "Acquisition:Binary Sample Width", "Actual Sample Rate", "Actual Record Length"](reference=w1156, error in=w1157, "Fetch:Fetch Relative To"=w1155) -> (reference out=w1149:refnum<k15>, error out=w1148:errorcluster, "Actual Sample Rate"=→"Sample Rate IND":dbl)  [unwired: 2 out]
                  }
                }
                n437 = Divide(x=15000000.0, y=w1034) -> (x/y=w1032:dbl)
                n438 = To Long Integer(number=w1032) -> (32bit integer=w1031:i32)
                n439 = Concatenate Strings(w1048) -> (w1047:string)
              }
              frame "CONFIGSCOPE" {
                n440 = flat-sequence {
                  tunnel: w1188 -> [w1210]
                  tunnel: w1193 -> [w1211]
                  tunnel: w1198 -> [w1212]
                  tunnel: w1201 -> [w1213]
                  tunnel: w1202 -> [w1214]
                  tunnel: w1203 -> [w1206]
                  tunnel: w1204 -> [w1215]
                  tunnel: [w1215] -> w1184
                  tunnel: [w1214] -> w1182
                  tunnel: [w1213] -> w1180
                  tunnel: [w1212] -> w1178
                  tunnel: [w1211] -> w1176
                  tunnel: [w1207] -> w1174
                  tunnel: [w1205] -> w1171
                  tunnel: w1184 -> [w1277]
                  tunnel: [w1277] -> w1183
                  tunnel: w1182 -> [w1276]
                  tunnel: [w1276] -> w1181
                  tunnel: w1180 -> [w1275]
                  tunnel: [w1275] -> w1179
                  tunnel: w1178 -> [w1274]
                  tunnel: [w1274] -> w1177
                  tunnel: w1176 -> [w1273]
                  tunnel: [w1273] -> w1175
                  tunnel: w1174 -> [w1272]
                  tunnel: [w1272] -> w1173
                  tunnel: [w1271] -> w1172
                  tunnel: w1171 -> [w1271]
                  tunnel: ["HOLDBY"] -> w1200
                  tunnel: w1197 -> [w1298]
                  tunnel: [w1294] -> w1196
                  tunnel: [w1293] -> w1195
                  tunnel: w1194 -> [w1288]
                  tunnel: [w1282] -> w1187
                  tunnel: w1183 -> [w1313]
                  tunnel: w1181 -> [w1312]
                  tunnel: w1179 -> [w1311]
                  tunnel: w1177 -> [w1299]
                  tunnel: w1175 -> [w1287]
                  tunnel: w1173 -> [w1278]
                  tunnel: w1172 -> [w1279]
                  tunnel: [w1278] -> w1170
                  frame #0 {
                    n441 = while {
                      shift-right: [w1231] -> _
                      shift-left: w1210 -> [w1232]
                      shift-right: [w1217] -> _
                      shift-left: 0 -> [w1223]
                      shift-right: [w1225] -> w1207
                      shift-left: "" -> [w1221]
                      tunnel: [w1231] -> _ mode=indexing
                      tunnel: w1206 -> [w1220]
                      tunnel: [w1219] -> w1205
                      i -> [w1230]
                      stop <- w1229 stop-if-true
                      n442 = flat-sequence {
                        tunnel: w1232 -> [w1242]
                        tunnel: w1230 -> [_]
                        tunnel: [w1240] -> w1228
                        tunnel: [w1233] -> w1227
                        tunnel: [w1234] -> w1226
                        tunnel: [w1239] -> w1224
                        tunnel: w1223 -> [w1239]
                        tunnel: [w1238] -> w1222
                        tunnel: w1221 -> [w1238]
                        tunnel: [w1233] -> w1216
                        tunnel: w1228 -> [w1254]
                        tunnel: w1227 -> [w1245]
                        tunnel: w1226 -> [w1253]
                        tunnel: w1224 -> [w1251]
                        tunnel: w1222 -> [w1250]
                        tunnel: w1220 -> [w1249]
                        tunnel: [w1254] -> w1231
                        tunnel: [w1245] -> w1229
                        tunnel: [w1252] -> w1225
                        tunnel: [w1248] -> w1219
                        tunnel: [w1247] -> w1218
                        tunnel: w1216 -> [w1246]
                        frame #0 {
                          n443 = Match Pattern(string=w1242, regular expression=",") -> (before substring=w1237:string, after substring=w1240:string, offset past match=w1244:i32)  [unwired: 1 in, 1 out]
                          n444 = Equal?(x=w1237, y="") -> (x = y?=w1235:bool)
                          n445 = Equal?(x=w1244, y=-1) -> (x = y?=w1233:bool)
                          n446 = And(x=w1233, y=w1235) -> (x .and. y?=w1234:bool)
                        }
                        frame #1 {
                          n447 = case shown="False" w1253 {
                            tunnel: [w1255 ""] -> w1252
                            tunnel: w1251 -> [w1260 w1269]
                            tunnel: w1250 -> [w1258 _]
                            tunnel: [w1260 w1269] -> w1247
                            tunnel: w1249 -> [w1259 _]
                            tunnel: [w1259 errorcluster {"status"=TRUE, "code"=0, "source"="No Channel Parameter"} ("error out")] -> w1248
                            tunnel: w1246 -> [_ _]
                            tunnel: w1245 -> [w1256 _]
                            frame False {
                              n448 = Number To Decimal String(number=w1260) -> (decimal integer string=w1257:string)  [unwired: 1 in]
                              n449 = case shown="False" w1256 {
                                tunnel: w1258 -> [w1264 w1267]
                                tunnel: w1257 -> [w1263 w1266]
                                tunnel: [w1261 w1265] -> w1255
                                frame False {
                                n450 = Concatenate Strings(w1264, w1263, "," ("string")) -> (w1261:string)
                                }
                                frame True {
                                n451 = Concatenate Strings(w1267, w1266) -> (w1265:string)
                                }
                              }
                            }
                            frame True {
                            }
                          }
                        }
                      }
                      n452 = Increment(x=w1218) -> (x+1=w1217:i32)
                    }
                  }
                  frame #1 {
                  }
                  frame #2 {
                    w1295 = 388 items=["Start"=482, "Trigger"=483, "Pretrigger"=477, "Now"=481, "Read Pointer"=388] ("Fetch:Fetch Relative To")
                    w1314 = u32 0 items=["1 mega ohm"=0, "50 ohms"=2] ("input impedance")
                    # "3"
                    n453 = String Length(string=w1278) -> (length=w1286:i32)
                    n454 = call <instrlib>:"niScope Configure Vertical.vi"("instrument handle"=w1313, "vertical coupling"=w1287, "channels"=w1278, "vertical range"=w1311, "error in"=w1279) -> ("instrument handle out"=w1316:refnum<k15>, "error out"=w1315:errorcluster)  [unwired: 9 in]
                    n455 = Match Pattern(string=w1278, regular expression="0") -> (offset past match=w1301:i32)  [unwired: 1 in, 3 out]
                    n456 = Quotient & Remainder(x=w1286, y=2) -> (x-y*floor(x/y)=w1283:i32, floor(x/y)=w1284:i32)
                    n457 = Not Equal?(x=w1301, y=-1) -> (x != y?=w1302:bool)
                    n458 = And(x=w1299, y=w1302) -> (x .and. y?=w1303:bool)
                    n459 = Add(x=w1283, y=w1284) -> (x+y=w1282:i32)
                    n460 = call <instrlib>:"niScope Configure Chan Characteristics.vi"("instrument handle"=w1316, "channels"=w1278, "input impedance"=w1314, "maximum input frequency"=0.0, "error in"=w1315) -> ("instrument handle out"=w1306:refnum<k15>, "error out"=w1305:errorcluster)  [unwired: 9 in]
                    n461 = case shown="False" w1303 {
                      tunnel: [w1318 w1328] -> w1308
                      tunnel: [w1317 w1327] -> w1307
                      tunnel: w1306 -> [w1318 w1322]
                      tunnel: w1305 -> [w1317 w1321]
                      tunnel: w1298 -> [_ w1319]
                      frame False {
                      }
                      frame True {
                        w1325 = u32 2 items=["1 mega ohm"=0, "50 ohms"=2] ("input impedance")
                        w1320 = "0" ("channels")
                        n462 = call <instrlib>:"niScope Configure Vertical.vi"("instrument handle"=w1322, "channels"=w1320, "vertical range"=w1319, "error in"=w1321) -> ("instrument handle out"=w1324:refnum<k15>, "error out"=w1323:errorcluster)  [unwired: 10 in]
                        n463 = call <instrlib>:"niScope Configure Chan Characteristics.vi"("instrument handle"=w1324, "channels"=w1320, "input impedance"=w1325, "maximum input frequency"=0.0, "error in"=w1323) -> ("instrument handle out"=w1328:refnum<k15>, "error out"=w1327:errorcluster)  [unwired: 9 in]
                      }
                    }
                    n464 = call <instrlib>:"niScope Configure Horizontal Timing.vi"("instrument handle"=w1308, "min sample rate"=w1312, "error in"=w1307, "min record length"=w1288) -> ("instrument handle out"=w1280:refnum<k15>, "error out"=w1281:errorcluster)  [unwired: 10 in]
                    n465 = call-poly <instrlib>:"niScope Configure Trigger (poly).vi"("instrument handle"=w1280, "error in"=w1281) -> ("instrument handle out"=w1290:refnum<k15>, "error out"=w1289:errorcluster)  [unwired: 12 in]
                    n466 = call <instrlib>:"niScope Initiate Acquisition.vi"("instrument handle"=w1290, "error in"=w1289) -> ("instrument handle out"=w1296:refnum<k15>, "error out"=w1297:errorcluster)  [unwired: 12 in]
                    n467 = property class="niScope" props=["Fetch:Fetch Relative To", "Acquisition:Binary Sample Width"](reference=w1296, error in=w1297, "Fetch:Fetch Relative To"=w1295) -> (reference out=w1291:refnum<k15>, error out=w1292:errorcluster)  [unwired: 1 out]
                    n468 = call <instrlib>:"niScope Abort.vi"("instrument handle"=w1291, "error in"=w1292) -> ("instrument handle out"=w1294:refnum<k15>, "error out"=w1293:errorcluster)  [unwired: 12 in]
                  }
                }
                n469 = Concatenate Strings(w1200) -> (w1199:string)
              }
              frame "WAIT4FOLDER" {
                n470 = local read "FOLDERCREATED"() -> (w1338:bool)
                n471 = case shown="True" w1338 {
                  tunnel: [w1347 w1357] -> w1344
                  tunnel: w1343 -> [w1347 w1359]
                  tunnel: w1342 -> [w1346 w1358]
                  tunnel: [w1346 w1356] -> w1341
                  tunnel: w1340 -> [w1345 _]
                  tunnel: [w1345 w1355] -> w1339
                  tunnel: w1330 -> [_ w1349]
                  tunnel: w1329 -> [_ w1348]
                  frame False {
                  }
                  frame True {
                    n472 = flat-sequence {
                      tunnel: w1358 -> [w1362]
                      tunnel: w1359 -> [w1363]
                      tunnel: [w1363] -> w1351
                      tunnel: [w1362] -> w1350
                      tunnel: w1349 -> [w1361]
                      tunnel: w1348 -> [w1360]
                      tunnel: [w1468] -> w1354
                      tunnel: [w1467] -> w1353
                      tunnel: [w1463] -> w1352
                      tunnel: w1351 -> [w1470]
                      tunnel: w1350 -> [w1469]
                      tunnel: [w1472] -> w1355
                      tunnel: [w1473] -> w1356
                      tunnel: [w1474] -> w1357
                      tunnel: w1354 -> [w1474]
                      tunnel: w1353 -> [w1473]
                      tunnel: w1352 -> [w1472]
                      frame #0 {
                        n473 = case shown="2" w1360 {
                          tunnel: w1361 -> [_ w1365 w1370 w1378 w1388 w1399 w1405 w1421 w1445 _]
                          frame ..0 {
                          }
                          frame 1, Default {
                            w1364 = "CHANNEL_NOT_DEFINED" ("CHANNEL 3 NAME")
                            n474 = local write "CHANNEL 0 NAME"(w1365) -> ()
                            n475 = local write "CHANNEL 1 NAME"(w1364) -> ()
                            n476 = local write "CHANNEL 3 NAME"(w1364) -> ()
                            n477 = local write "CHANNEL 4 NAME"(w1364) -> ()
                            n478 = local write "CHANNEL 5 NAME"(w1364) -> ()
                            n479 = local write "CHANNEL 6 NAME"(w1364) -> ()
                            n480 = local write "CHANNEL 7 NAME"(w1364) -> ()
                            n481 = local write "CHANNEL 2 NAME"(w1364) -> ()
                          }
                          frame 2 {
                            w1366 = "CHANNEL_NOT_DEFINED" ("CHANNEL 3 NAME")
                            n482 = Match Pattern(string=w1370, regular expression=",") -> (before substring=w1368:string, after substring=w1367:string)  [unwired: 1 in, 2 out]
                            n483 = local write "CHANNEL 0 NAME"(w1368) -> ()
                            n484 = local write "CHANNEL 1 NAME"(w1367) -> ()
                            n485 = local write "CHANNEL 2 NAME"(w1366) -> ()
                            n486 = local write "CHANNEL 4 NAME"(w1366) -> ()
                            n487 = local write "CHANNEL 5 NAME"(w1366) -> ()
                            n488 = local write "CHANNEL 6 NAME"(w1366) -> ()
                            n489 = local write "CHANNEL 7 NAME"(w1366) -> ()
                            n490 = local write "CHANNEL 3 NAME"(w1366) -> ()
                          }
                          frame 3 {
                            w1371 = "CHANNEL_NOT_DEFINED" ("CHANNEL 3 NAME")
                            n491 = Match Pattern(string=w1378, regular expression=",") -> (before substring=w1376:string, after substring=w1374:string)  [unwired: 1 in, 2 out]
                            n492 = local write "CHANNEL 0 NAME"(w1376) -> ()
                            n493 = Match Pattern(string=w1374, regular expression=",") -> (before substring=w1373:string, after substring=w1372:string)  [unwired: 1 in, 2 out]
                            n494 = local write "CHANNEL 1 NAME"(w1373) -> ()
                            n495 = local write "CHANNEL 2 NAME"(w1372) -> ()
                            n496 = local write "CHANNEL 3 NAME"(w1371) -> ()
                            n497 = local write "CHANNEL 5 NAME"(w1371) -> ()
                            n498 = local write "CHANNEL 6 NAME"(w1371) -> ()
                            n499 = local write "CHANNEL 7 NAME"(w1371) -> ()
                            n500 = local write "CHANNEL 4 NAME"(w1371) -> ()
                          }
                          frame 4 {
                            w1379 = "CHANNEL_NOT_DEFINED" ("CHANNEL 3 NAME")
                            n501 = Match Pattern(string=w1388, regular expression=",") -> (before substring=w1387:string, after substring=w1385:string)  [unwired: 1 in, 2 out]
                            n502 = local write "CHANNEL 0 NAME"(w1387) -> ()
                            n503 = Match Pattern(string=w1385, regular expression=",") -> (before substring=w1384:string, after substring=w1381:string)  [unwired: 1 in, 2 out]
                            n504 = local write "CHANNEL 1 NAME"(w1384) -> ()
                            n505 = Match Pattern(string=w1381, regular expression=",") -> (before substring=w1382:string, after substring=w1380:string)  [unwired: 1 in, 2 out]
                            n506 = local write "CHANNEL 2 NAME"(w1382) -> ()
                            n507 = local write "CHANNEL 3 NAME"(w1380) -> ()
                            n508 = local write "CHANNEL 4 NAME"(w1379) -> ()
                            n509 = local write "CHANNEL 6 NAME"(w1379) -> ()
                            n510 = local write "CHANNEL 7 NAME"(w1379) -> ()
                            n511 = local write "CHANNEL 5 NAME"(w1379) -> ()
                          }
                          frame 5 {
                            w1390 = "CHANNEL_NOT_DEFINED" ("CHANNEL 3 NAME")
                            n512 = Match Pattern(string=w1399, regular expression=",") -> (before substring=w1397:string, after substring=w1398:string)  [unwired: 1 in, 2 out]
                            n513 = local write "CHANNEL 0 NAME"(w1397) -> ()
                            n514 = Match Pattern(string=w1398, regular expression=",") -> (before substring=w1396:string, after substring=w1395:string)  [unwired: 1 in, 2 out]
                            n515 = local write "CHANNEL 1 NAME"(w1396) -> ()
                            n516 = Match Pattern(string=w1395, regular expression=",") -> (before substring=w1394:string, after substring=w1393:string)  [unwired: 1 in, 2 out]
                            n517 = local write "CHANNEL 2 NAME"(w1394) -> ()
                            n518 = Match Pattern(string=w1393, regular expression=",") -> (before substring=w1392:string, after substring=w1391:string)  [unwired: 1 in, 2 out]
                            n519 = local write "CHANNEL 5 NAME"(w1390) -> ()
                            n520 = local write "CHANNEL 7 NAME"(w1390) -> ()
                            n521 = local write "CHANNEL 6 NAME"(w1390) -> ()
                            n522 = local write "CHANNEL 3 NAME"(w1392) -> ()
                            n523 = local write "CHANNEL 4 NAME"(w1391) -> ()
                          }
                          frame 6 {
                            w1404 = "CHANNEL_NOT_DEFINED" ("CHANNEL 3 NAME")
                            n524 = Match Pattern(string=w1405, regular expression=",") -> (before substring=w1415:string, after substring=w1414:string)  [unwired: 1 in, 2 out]
                            n525 = local write "CHANNEL 0 NAME"(w1415) -> ()
                            n526 = Match Pattern(string=w1414, regular expression=",") -> (before substring=w1413:string, after substring=w1411:string)  [unwired: 1 in, 2 out]
                            n527 = local write "CHANNEL 1 NAME"(w1413) -> ()
                            n528 = Match Pattern(string=w1411, regular expression=",") -> (before substring=w1412:string, after substring=w1410:string)  [unwired: 1 in, 2 out]
                            n529 = local write "CHANNEL 2 NAME"(w1412) -> ()
                            n530 = Match Pattern(string=w1410, regular expression=",") -> (before substring=w1409:string, after substring=w1408:string)  [unwired: 1 in, 2 out]
                            n531 = local write "CHANNEL 6 NAME"(w1404) -> ()
                            n532 = local write "CHANNEL 7 NAME"(w1404) -> ()
                            n533 = local write "CHANNEL 3 NAME"(w1409) -> ()
                            n534 = Match Pattern(string=w1408, regular expression=",") -> (before substring=w1406:string, after substring=w1407:string)  [unwired: 1 in, 2 out]
                            n535 = local write "CHANNEL 4 NAME"(w1406) -> ()
                            n536 = local write "CHANNEL 5 NAME"(w1407) -> ()
                          }
                          frame 8 {
                            n537 = Match Pattern(string=w1421, regular expression=",") -> (before substring=w1435:string, after substring=w1434:string)  [unwired: 1 in, 2 out]
                            n538 = local write "CHANNEL 0 NAME"(w1435) -> ()
                            n539 = Match Pattern(string=w1434, regular expression=",") -> (before substring=w1433:string, after substring=w1432:string)  [unwired: 1 in, 2 out]
                            n540 = local write "CHANNEL 1 NAME"(w1433) -> ()
                            n541 = Match Pattern(string=w1432, regular expression=",") -> (before substring=w1431:string, after substring=w1430:string)  [unwired: 1 in, 2 out]
                            n542 = local write "CHANNEL 2 NAME"(w1431) -> ()
                            n543 = Match Pattern(string=w1430, regular expression=",") -> (before substring=w1429:string, after substring=w1428:string)  [unwired: 1 in, 2 out]
                            n544 = local write "CHANNEL 3 NAME"(w1429) -> ()
                            n545 = Match Pattern(string=w1428, regular expression=",") -> (before substring=w1427:string, after substring=w1426:string)  [unwired: 1 in, 2 out]
                            n546 = local write "CHANNEL 4 NAME"(w1427) -> ()
                            n547 = Match Pattern(string=w1426, regular expression=",") -> (before substring=w1425:string, after substring=w1424:string)  [unwired: 1 in, 2 out]
                            n548 = local write "CHANNEL 5 NAME"(w1425) -> ()
                            n549 = Match Pattern(string=w1424, regular expression=",") -> (before substring=w1423:string, after substring=w1422:string)  [unwired: 1 in, 2 out]
                            n550 = local write "CHANNEL 6 NAME"(w1423) -> ()
                            n551 = local write "CHANNEL 7 NAME"(w1422) -> ()
                          }
                          frame 7 {
                            n552 = Match Pattern(string=w1445, regular expression=",") -> (before substring=w1456:string, after substring=w1455:string)  [unwired: 1 in, 2 out]
                            n553 = local write "CHANNEL 0 NAME"(w1456) -> ()
                            n554 = Match Pattern(string=w1455, regular expression=",") -> (before substring=w1454:string, after substring=w1453:string)  [unwired: 1 in, 2 out]
                            n555 = local write "CHANNEL 1 NAME"(w1454) -> ()
                            n556 = Match Pattern(string=w1453, regular expression=",") -> (before substring=w1452:string, after substring=w1451:string)  [unwired: 1 in, 2 out]
                            n557 = local write "CHANNEL 2 NAME"(w1452) -> ()
                            n558 = Match Pattern(string=w1451, regular expression=",") -> (before substring=w1450:string, after substring=w1449:string)  [unwired: 1 in, 2 out]
                            n559 = local write "CHANNEL 7 NAME"("CHANNEL_NOT_DEFINED" ("CHANNEL 3 NAME")) -> ()
                            n560 = local write "CHANNEL 3 NAME"(w1450) -> ()
                            n561 = Match Pattern(string=w1449, regular expression=",") -> (before substring=w1448:string, after substring=w1447:string)  [unwired: 1 in, 2 out]
                            n562 = local write "CHANNEL 4 NAME"(w1448) -> ()
                            n563 = Match Pattern(string=w1447, regular expression=",") -> (before substring=w1446:string, after substring=w1444:string)  [unwired: 1 in, 2 out]
                            n564 = local write "CHANNEL 5 NAME"(w1446) -> ()
                            n565 = local write "CHANNEL 6 NAME"(w1444) -> ()
                          }
                          frame 9.. {
                          }
                        }
                      }
                      frame #1 {
                        n566 = property class="niScope"(reference=w1470, error in=w1469) -> (reference out=w1468:refnum<k15>, error out=w1467:errorcluster, "Acquisition:Binary Sample Width"=w1465:i32)
                        n567 = Number To Decimal String(number=w1465) -> (decimal integer string=w1464:string)  [unwired: 1 in]
                        n568 = Concatenate Strings("COLLECTION", w1464) -> (w1463:string)
                      }
                      frame #2 {
                        n569 = local write "FOLDERCREATED"(FALSE) -> ()
                      }
                    }
                  }
                }
              }
              frame "COLLECTION16" {
                n570 = case shown="True" w1497 {
                  tunnel: w1502 -> [w1512 w1603]
                  tunnel: w1501 -> [w1511 w1602]
                  tunnel: [w1509 w1600] -> w1500
                  tunnel: [w1510 w1595] -> w1499
                  tunnel: ["HOLDOFF" w1516] -> w1498
                  tunnel: w1496 -> [_ w1516]
                  tunnel: w1495 -> [_ _]
                  tunnel: w1494 -> [_ w1601]
                  tunnel: w1493 -> [_ w1549]
                  tunnel: w1492 -> [w1507 w1594]
                  tunnel: w1491 -> [_ w1591]
                  tunnel: w1490 -> [_ w1589]
                  tunnel: w1489 -> [_ w1587]
                  tunnel: w1488 -> [w1505 w1585]
                  tunnel: w1487 -> [w1506 w1583]
                  tunnel: w1486 -> [w1508 w1581]
                  tunnel: [w1508 w1580] -> w1485
                  tunnel: [w1506 w1579] -> w1484
                  tunnel: [w1507 w1578] -> w1483
                  tunnel: [w1505 w1577] -> w1482
                  tunnel: w1481 -> [_ w1575]
                  tunnel: [w1504 w1574] -> w1480
                  tunnel: w1479 -> [w1504 w1572]
                  tunnel: w1478 -> [_ w1517]
                  tunnel: w1477 -> [_ w1518]
                  tunnel: [w1503 w1515] -> w1476
                  tunnel: w1475 -> [w1503 w1515]
                  frame False {
                    n571 = call <instrlib>:"niScope Abort.vi"("instrument handle"=w1512, "error in"=w1511) -> ("instrument handle out"=w1510:refnum<k15>, "error out"=w1509:errorcluster)  [unwired: 12 in]
                  }
                  frame True {
                    n572 = flat-sequence {
                      tunnel: w1601 -> [w1622]
                      tunnel: [w1604] -> _
                      tunnel: w1602 -> [w1623]
                      tunnel: w1603 -> [w1624]
                      tunnel: [w1624] -> w1599
                      tunnel: [w1623] -> w1598
                      tunnel: [w1604] -> w1597
                      tunnel: [w1622] -> w1596
                      tunnel: w1594 -> [w1620]
                      tunnel: [w1620] -> w1593
                      tunnel: [w1619] -> w1592
                      tunnel: w1591 -> [w1619]
                      tunnel: [w1618] -> w1590
                      tunnel: w1589 -> [w1618]
                      tunnel: [w1617] -> w1588
                      tunnel: w1587 -> [w1617]
                      tunnel: [w1616] -> w1586
                      tunnel: w1585 -> [w1616]
                      tunnel: [w1615] -> w1584
                      tunnel: w1583 -> [w1615]
                      tunnel: [w1614] -> w1582
                      tunnel: w1581 -> [w1614]
                      tunnel: [w1613] -> w1576
                      tunnel: w1575 -> [w1613]
                      tunnel: w1572 -> [w1612]
                      tunnel: [w1612] -> w1573
                      tunnel: w1517 -> [w1607]
                      tunnel: [w1606] -> w1519
                      tunnel: w1518 -> [w1605]
                      tunnel: w1515 -> [w1604]
                      tunnel: w1599 -> [w1642]
                      tunnel: w1598 -> [w1641]
                      tunnel: w1597 -> [w1640]
                      tunnel: w1596 -> [w1639]
                      tunnel: [w1628] -> w1548
                      tunnel: [w1638] -> w1546
                      tunnel: [w1626] -> w1544
                      tunnel: [w1627] -> w1542
                      tunnel: w1593 -> [w1637]
                      tunnel: [w1637] -> w1540
                      tunnel: [w1636] -> w1538
                      tunnel: w1592 -> [w1636]
                      tunnel: [w1635] -> w1536
                      tunnel: w1590 -> [w1635]
                      tunnel: [w1634] -> w1534
                      tunnel: w1588 -> [w1634]
                      tunnel: w1586 -> [w1633]
                      tunnel: [w1633] -> w1532
                      tunnel: [w1632] -> w1530
                      tunnel: w1584 -> [w1632]
                      tunnel: [w1631] -> w1528
                      tunnel: w1582 -> [w1631]
                      tunnel: w1576 -> [w1630]
                      tunnel: [w1630] -> w1526
                      tunnel: w1573 -> [w1629]
                      tunnel: [w1629] -> w1524
                      tunnel: [w1626] -> w1522
                      tunnel: [w1625] -> w1520
                      tunnel: w1519 -> [w1625]
                      tunnel: w1548 -> [w1661]
                      tunnel: [w1661] -> w1547
                      tunnel: w1546 -> [w1660]
                      tunnel: [w1660] -> w1545
                      tunnel: w1544 -> [w1659]
                      tunnel: [w1659] -> w1543
                      tunnel: w1542 -> [w1658]
                      tunnel: [w1658] -> w1541
                      tunnel: w1540 -> [w1657]
                      tunnel: [w1657] -> w1539
                      tunnel: w1538 -> [w1656]
                      tunnel: [w1656] -> w1537
                      tunnel: w1536 -> [w1655]
                      tunnel: [w1655] -> w1535
                      tunnel: w1534 -> [w1654]
                      tunnel: [w1654] -> w1533
                      tunnel: w1532 -> [w1653]
                      tunnel: [w1653] -> w1531
                      tunnel: w1530 -> [w1652]
                      tunnel: [w1652] -> w1529
                      tunnel: w1528 -> [w1651]
                      tunnel: [w1651] -> w1527
                      tunnel: w1526 -> [w1650]
                      tunnel: [w1650] -> w1525
                      tunnel: w1524 -> [w1647]
                      tunnel: [w1648] -> w1523
                      tunnel: w1522 -> [w1649]
                      tunnel: [w1649] -> w1521
                      tunnel: w1520 -> [w1646]
                      tunnel: [w1644] -> w1514
                      tunnel: w1547 -> [w1714]
                      tunnel: w1545 -> [w1713]
                      tunnel: w1543 -> [w1682]
                      tunnel: w1541 -> [w1678]
                      tunnel: w1539 -> [w1693]
                      tunnel: w1537 -> [w1691]
                      tunnel: w1535 -> [w1690]
                      tunnel: w1533 -> [w1692]
                      tunnel: w1531 -> [w1689]
                      tunnel: w1529 -> [w1687]
                      tunnel: w1527 -> [w1688]
                      tunnel: [w1714] -> w1571
                      tunnel: [w1713] -> w1569
                      tunnel: [w1686] -> w1567
                      tunnel: [w1685] -> w1565
                      tunnel: [w1684] -> w1563
                      tunnel: [w1683] -> w1561
                      tunnel: [w1678] -> w1559
                      tunnel: [w1682] -> w1557
                      tunnel: [w1681] -> w1555
                      tunnel: w1525 -> [w1681]
                      tunnel: [w1680] -> w1553
                      tunnel: w1523 -> [w1680]
                      tunnel: [w1679] -> w1551
                      tunnel: w1521 -> [w1679]
                      tunnel: [w1678] -> w1550
                      tunnel: w1514 -> [w1674]
                      tunnel: w1571 -> [w1791]
                      tunnel: [w1790] -> w1570
                      tunnel: w1569 -> [w1799]
                      tunnel: [w1799] -> w1568
                      tunnel: w1567 -> [w1798]
                      tunnel: [w1798] -> w1566
                      tunnel: w1565 -> [w1797]
                      tunnel: [w1797] -> w1564
                      tunnel: w1563 -> [w1786]
                      tunnel: [w1786] -> w1562
                      tunnel: w1561 -> [w1796]
                      tunnel: [w1796] -> w1560
                      tunnel: w1559 -> [w1795]
                      tunnel: [w1795] -> w1558
                      tunnel: w1557 -> [w1794]
                      tunnel: [w1794] -> w1556
                      tunnel: w1555 -> [w1793]
                      tunnel: [w1793] -> w1554
                      tunnel: w1553 -> [w1792]
                      tunnel: [w1792] -> w1552
                      tunnel: w1551 -> [w1789]
                      tunnel: w1550 -> [w1788]
                      tunnel: w1549 -> [w1783]
                      tunnel: [w1808] -> w1577
                      tunnel: [w1809] -> w1578
                      tunnel: [w1810] -> w1579
                      tunnel: [w1811] -> w1580
                      tunnel: [w1812] -> w1595
                      tunnel: [w1803] -> w1600
                      tunnel: w1570 -> [w1807]
                      tunnel: w1568 -> [w1812]
                      tunnel: w1566 -> [w1811]
                      tunnel: w1564 -> [w1810]
                      tunnel: w1562 -> [w1809]
                      tunnel: w1560 -> [w1808]
                      tunnel: w1558 -> [w1806]
                      tunnel: w1556 -> [w1805]
                      tunnel: w1554 -> [w1804]
                      tunnel: [w1802] -> w1574
                      tunnel: w1552 -> [w1801]
                      frame #0 {
                        n573 = Quotient & Remainder(x=w1607, y=w1605) -> (x-y*floor(x/y)=w1610:i32, floor(x/y)=w1611:i32)
                        n574 = Equal To 0?(x=w1610) -> (x = 0?=w1609:bool)
                        n575 = Not Equal To 0?(x=w1611) -> (x != 0?=w1608:bool)
                        n576 = And(x=w1609, y=w1608) -> (x .and. y?=w1606:bool)
                        n577 = Wait (ms)(milliseconds to wait="milliseconds to wait") -> ()  [unwired: 1 out]
                      }
                      frame #1 {
                        w1643 = 0.0  # timeout
                        n578 = call-poly <instrlib>:"niScope Fetch (poly).vi"("timeout"=w1643, "error in"=w1641, "numSamples"=w1639, "channels"=w1640, "instrument handle"=w1642) -> ("error out"=w1628:errorcluster, "wfm"=w1627:i16[][], "wfm info"=w1626:T3, "instrument handle out"=w1638:refnum<k15>)  [unwired: 3 in]
                        "wfm info IND" <- w1626
                      }
                      frame #2 {
                        n579 = case shown="True" w1646 {
                          tunnel: [w1662 w1663] -> w1648
                          tunnel: w1647 -> [w1662 _]
                          frame False {
                          }
                          frame True {
                            n580 = Bundle("array"=dbl[] [], "array"=dbl[] [], "array"=dbl[] [], "array"=dbl[] [], "array"=dbl[] [], "array"=dbl[] [], "array"=dbl[] [], "array"=dbl[] []) -> (w1663:T7)  [unwired: 1 in]
                          }
                        }
                        n581 = local read "IndicatorOutputs"() -> (w1645:cluster{"Run Information":string, string})
                        n582 = Unbundle(w1645) -> (w1644:string)  [unwired: 1 out]
                      }
                      frame #3 {
                        # "shift register"
                        # "SHIFT REGISTER"
                        n583 = Increment(x=w1690) -> (x+1=w1703:dbl)
                        n584 = Negate(x=w1690) -> (-x=w1702:dbl)
                        n585 = Index Array(array=w1678, index (row)=0 ("index")) -> (element=w1696:i16[])  [unwired: 1 in]
                        n586 = Multiply(x=w1691, y=w1703) -> (x*y=w1673:dbl)
                        n587 = Increment(x=w1702) -> (x+1=w1701:dbl)
                        n588 = Array Size(array=w1696) -> (size(s)=w1695:i32)
                        "Last Point Fetched" <- w1695
                        n589 = Add(x=w1695, y=w1693) -> (x+y=→"Total Points Fetched":i32)
                        n590 = Multiply(x=w1691, y=w1701) -> (x*y=w1676:dbl)
                        n591 = Index Array(array=w1682, index="Channel To Mitigate (0-7)") -> (element=w1712:T12)
                        n592 = Index Array(array=w1678, index (row)="Channel To Mitigate (0-7)") -> (element=w1709:i16[])  [unwired: 1 in]
                        n593 = Unbundle By Name(w1712) -> ("actualSamples"=→"NUMBER SAMPLES":i32, "xIncrement"=→"XINC":dbl, "absoluteInitialX"=w1711:dbl)
                        n594 = Unbundle By Name(w1712) -> ("gain"=w1707:dbl, "offset"=w1705:dbl)
                        n595 = To Double Precision Float(number=w1709) -> (double precision float=w1708:dbl[])
                        n596 = Multiply(x=w1707, y=w1708) -> (x*y=w1706:dbl[])
                        n597 = Add(x=w1705, y=w1706) -> (x+y=w1704:dbl[])
                        n598 = case shown="\"Latchup\", Default" w1674 {
                          tunnel: w1704 -> [w1716 w1724]
                          tunnel: [w1717 w1722] -> w1677
                          tunnel: w1676 -> [_ w1720]
                          tunnel: [w1718 w1721] -> w1675
                          tunnel: w1673 -> [w1715 _]
                          tunnel: [w1715 w1720] -> w1672
                          frame "Latchup", Default {
                            n599 = Array Max & Min(array=w1716) -> (max value=w1719:dbl, max index (indices)=w1717:i32)  [unwired: 2 out]
                            n600 = Greater?(x=w1719, y=w1715) -> (0:w1718:bool)
                          }
                          frame "Transient" {
                            # "shift register"
                            n601 = Array Max & Min(array=w1724) -> (min value=w1723:dbl, min index (indices)=w1722:i32)  [unwired: 2 out]
                            n602 = Greater?(x=w1720, y=w1723) -> (0:w1721:bool)
                          }
                        }
                        "EXCEED THRESHOLD" <- w1675
                        "Threshold Value" <- w1672
                        n603 = disable-structure shown="Enabled" {
                          disable-tunnel: w1675 -> [w1736 w1782]
                          disable-tunnel: w1711 -> [w1735 _]
                          disable-tunnel: [w1734 w1782] -> w1710
                          disable-tunnel: w1692 -> [w1733 _]
                          disable-tunnel: w1689 -> [w1732 w1781]
                          disable-tunnel: w1688 -> [w1731 _]
                          disable-tunnel: w1687 -> [w1730 _]
                          disable-tunnel: [w1729 _] -> w1686
                          disable-tunnel: [w1728 _] -> w1685
                          disable-tunnel: [w1727 w1780] -> w1684
                          disable-tunnel: [w1726 w1781] -> w1683
                          disable-tunnel: w1677 -> [w1725 w1780]
                          frame Enabled {
                            n604 = case shown="True" w1736 {
                              selector: w1736 -> [w1740 w1754]
                              tunnel: w1732 -> [w1737 w1745]
                              tunnel: w1725 -> [_ w1743]
                              tunnel: [-1 w1742] -> w1727
                              tunnel: w1735 -> [_ w1750]
                              tunnel: w1731 -> [_ w1752]
                              tunnel: [w1740 w1754] -> w1729
                              tunnel: [0.0 w1749] -> w1728
                              tunnel: w1730 -> [_ w1748]
                              tunnel: w1733 -> [_ w1747]
                              tunnel: [FALSE w1746] -> w1734
                              tunnel: [w1737 w1744] -> w1726
                              frame False {
                              }
                              frame True {
                                n605 = Not(x=w1752) -> (.not. x?=w1753:bool)
                                n606 = And(x=w1753, y=w1754) -> (x .and. y?=w1751:bool)
                                n607 = case shown="False" w1751 {
                                tunnel: w1750 -> [w1765 w1779]
                                tunnel: [w1761 w1778] -> w1749
                                tunnel: w1748 -> [w1755 _]
                                tunnel: w1747 -> [w1763 _]
                                tunnel: [w1760 FALSE] -> w1746
                                tunnel: w1745 -> [w1759 w1776]
                                tunnel: [w1758 w1776] -> w1744
                                tunnel: [w1757 -1] -> w1742
                                tunnel: w1743 -> [w1756 _]
                                frame False {
                                n608 = Add(x=w1755, y=w1765) -> (x+y=w1762:dbl)
                                n609 = Greater?(x=w1762, y=w1763) -> (0:w1764:bool)
                                n610 = case shown="True" w1764 {
                                selector: w1764 -> [w1769 w1773]
                                tunnel: w1762 -> [_ _]
                                tunnel: [w1766 0.0] -> w1761
                                tunnel: [w1769 w1773] -> w1760
                                tunnel: w1759 -> [w1768 w1772]
                                tunnel: [w1768 w1771] -> w1758
                                tunnel: [-1 w1770] -> w1757
                                tunnel: w1756 -> [_ w1770]
                                tunnel: w1755 -> [w1766 _]
                                frame False {
                                }
                                frame True {
                                n611 = Increment(x=w1772) -> (x+1=w1771:i32)
                                }
                                }
                                }
                                frame True {
                                n612 = Negate(x=w1779) -> (-x=w1778:dbl)
                                }
                                }
                              }
                            }
                          }
                          frame Disabled {
                          }
                        }
                        "Over Threshold Number" <- w1683
                        "EXCEED DURATION" <- w1710
                        "Percent Threshold IND" <- w1690
                        "Nominal Current IND" <- w1691
                        "Channel To Mitigate (0-7) IND" <- "Channel To Mitigate (0-7)"
                      }
                      frame #4 {
                        (unwired) T11 {"wfm info"=[], "wfm"=[]} ("cluster")
                        n613 = Bundle(cluster=T8 {"wfm info"=[], "wfm"=[], "Beam On?"=FALSE, 0}, "wfm info"=w1789, "wfm"=w1788, "Beam On?"="Beam On?", w1786) -> (w1784:T8)
                        n614 = Enqueue Element(queue=w1783, element=w1784, error in (no error)=w1791) -> (error out=w1790:errorcluster)  [unwired: 1 in, 2 out]
                      }
                      frame #5 {
                        n615 = case shown="True" "Plot Data?" {
                          tunnel: w1804 -> [_ w1821]
                          tunnel: w1805 -> [_ w1820]
                          tunnel: w1806 -> [_ w1819]
                          tunnel: [w1814 w1818] -> w1803
                          tunnel: w1807 -> [w1814 w1817]
                          tunnel: [w1813 w1816] -> w1802
                          tunnel: w1801 -> [w1813 w1815]
                          frame False {
                          }
                          frame True {
                            n616 = case shown="8" w1821 {
                              tunnel: w1820 -> [_ w1838 w1860 w1885 w1913 w1947 w1983 w2025 w2070 _]
                              tunnel: w1819 -> [_ w1837 w1859 w1884 w1914 w1946 w1984 w2024 w2069 _]
                              tunnel: [w1823 w1836 w1858 w1883 w1912 w1945 w1982 w2023 w2068 w2090] -> w1818
                              tunnel: w1817 -> [w1823 w1836 w1858 w1883 w1912 w1945 w1982 w2023 w2068 w2090]
                              tunnel: [w1822 w1824 w1844 w1867 w1894 w1925 w1960 w2014 w2053 w2089] -> w1816
                              tunnel: w1815 -> [w1822 w1833 w1853 w1876 w1903 w1936 w1969 w2007 w2050 w2089]
                              frame ..0 {
                              }
                              frame 1, Default {
                                n617 = disable-structure shown="Enabled" {
                                disable-tunnel: 0 ("index") -> [w1841]
                                disable-tunnel: w1838 -> [w1842]
                                disable-tunnel: w1837 -> [w1840]
                                disable-tunnel: [w1843] -> w1835
                                frame Enabled {
                                n618 = call "StandAloneTransient_SingleGraphCreation_DataCollection_Light.vi"("wfm"=w1840, "index"=w1841, "wfm info"=w1842) -> ("Array"=w1843:dbl[])  [unwired: 8 in]
                                }
                                }
                                n619 = Unbundle(w1833) -> ("array"=w1832:dbl[], "array"=w1831:dbl[], "array"=w1830:dbl[], "array"=w1829:dbl[], "array"=w1828:dbl[], "array"=w1827:dbl[], "array"=w1826:dbl[], "array"=w1825:dbl[])
                                n620 = local write "Channel Graph 0"(w1835) -> ()
                                n621 = Insert Into Array(array=w1832, new element=w1835) -> (w1834:dbl[])  [unwired: 1 in]
                                n622 = local write "Channel Graph Cumulative 0"(w1834) -> ()
                                n623 = Bundle("array"=w1834, "array"=w1831, "array"=w1830, "array"=w1829, "array"=w1828, "array"=w1827, "array"=w1826, "array"=w1825) -> (w1824:T7)  [unwired: 1 in]
                              }
                              frame 2 {
                                n624 = disable-structure shown="Enabled" {
                                disable-tunnel: w1860 -> [w1863]
                                disable-tunnel: w1859 -> [w1864]
                                disable-tunnel: [w1862] -> w1857
                                disable-tunnel: [w1861] -> w1856
                                frame Enabled {
                                n625 = call "StandAloneTransient_SingleGraphCreation_DataCollection_Light.vi"("wfm"=w1864, "index"=0, "wfm info"=w1863) -> ("Array"=w1862:dbl[])  [unwired: 8 in]
                                n626 = call "StandAloneTransient_SingleGraphCreation_DataCollection_Light.vi"("wfm"=w1864, "index"=1, "wfm info"=w1863) -> ("Array"=w1861:dbl[])  [unwired: 8 in]
                                }
                                }
                                n627 = Unbundle(w1853) -> ("array"=w1852:dbl[], "array"=w1851:dbl[], "array"=w1850:dbl[], "array"=w1849:dbl[], "array"=w1848:dbl[], "array"=w1847:dbl[], "array"=w1846:dbl[], "array"=w1845:dbl[])
                                n628 = local write "Channel Graph 1"(w1856) -> ()
                                n629 = local write "Channel Graph 0"(w1857) -> ()
                                n630 = Insert Into Array(array=w1852, new element=w1856) -> (w1855:dbl[])  [unwired: 1 in]
                                n631 = Insert Into Array(array=w1851, new element=w1856) -> (w1854:dbl[])  [unwired: 1 in]
                                n632 = local write "Channel Graph Cumulative 0"(w1855) -> ()
                                n633 = local write "Channel Graph Cumulative 1"(w1854) -> ()
                                n634 = Bundle("array"=w1855, "array"=w1854, "array"=w1850, "array"=w1849, "array"=w1848, "array"=w1847, "array"=w1846, "array"=w1845) -> (w1844:T7)  [unwired: 1 in]
                              }
                              frame 3 {
                                n635 = disable-structure shown="Enabled" {
                                disable-tunnel: w1885 -> [w1890]
                                disable-tunnel: w1884 -> [w1889]
                                disable-tunnel: [w1893] -> w1882
                                disable-tunnel: [w1892] -> w1881
                                disable-tunnel: [w1891] -> w1880
                                frame Enabled {
                                n636 = call "StandAloneTransient_SingleGraphCreation_DataCollection_Light.vi"("wfm"=w1889, "index"=1, "wfm info"=w1890) -> ("Array"=w1892:dbl[])  [unwired: 8 in]
                                n637 = call "StandAloneTransient_SingleGraphCreation_DataCollection_Light.vi"("wfm"=w1889, "index"=2, "wfm info"=w1890) -> ("Array"=w1891:dbl[])  [unwired: 8 in]
                                n638 = call "StandAloneTransient_SingleGraphCreation_DataCollection_Light.vi"("wfm"=w1889, "index"=0, "wfm info"=w1890) -> ("Array"=w1893:dbl[])  [unwired: 8 in]
                                }
                                }
                                n639 = Unbundle(w1876) -> ("array"=w1875:dbl[], "array"=w1874:dbl[], "array"=w1873:dbl[], "array"=w1872:dbl[], "array"=w1871:dbl[], "array"=w1870:dbl[], "array"=w1869:dbl[], "array"=w1868:dbl[])
                                n640 = local write "Channel Graph 2"(w1880) -> ()
                                n641 = local write "Channel Graph 1"(w1881) -> ()
                                n642 = local write "Channel Graph 0"(w1882) -> ()
                                n643 = Insert Into Array(array=w1874, new element=w1881) -> (w1878:dbl[])  [unwired: 1 in]
                                n644 = Insert Into Array(array=w1873, new element=w1880) -> (w1877:dbl[])  [unwired: 1 in]
                                n645 = Insert Into Array(array=w1875, new element=w1882) -> (w1879:dbl[])  [unwired: 1 in]
                                n646 = local write "Channel Graph Cumulative 1"(w1878) -> ()
                                n647 = local write "Channel Graph Cumulative 2"(w1877) -> ()
                                n648 = local write "Channel Graph Cumulative 0"(w1879) -> ()
                                n649 = Bundle("array"=w1879, "array"=w1878, "array"=w1877, "array"=w1872, "array"=w1871, "array"=w1870, "array"=w1869, "array"=w1868) -> (w1867:T7)  [unwired: 1 in]
                              }
                              frame 4 {
                                n650 = disable-structure shown="Enabled" {
                                disable-tunnel: w1914 -> [w1924]
                                disable-tunnel: w1913 -> [w1923]
                                disable-tunnel: [w1915] -> w1911
                                disable-tunnel: [w1916] -> w1910
                                disable-tunnel: [w1917] -> w1909
                                disable-tunnel: [w1918] -> w1908
                                frame Enabled {
                                n651 = call "StandAloneTransient_SingleGraphCreation_DataCollection_Light.vi"("wfm"=w1924, "index"=2, "wfm info"=w1923) -> ("Array"=w1917:dbl[])  [unwired: 8 in]
                                n652 = call "StandAloneTransient_SingleGraphCreation_DataCollection_Light.vi"("wfm"=w1924, "index"=1, "wfm info"=w1923) -> ("Array"=w1916:dbl[])  [unwired: 8 in]
                                n653 = call "StandAloneTransient_SingleGraphCreation_DataCollection_Light.vi"("wfm"=w1924, "index"=3, "wfm info"=w1923) -> ("Array"=w1918:dbl[])  [unwired: 8 in]
                                n654 = call "StandAloneTransient_SingleGraphCreation_DataCollection_Light.vi"("wfm"=w1924, "index"=0, "wfm info"=w1923) -> ("Array"=w1915:dbl[])  [unwired: 8 in]
                                }
                                }
                                "Channel 0 Reference Values" <- w1911
                                n655 = Unbundle(w1903) -> ("array"=w1902:dbl[], "array"=w1901:dbl[], "array"=w1900:dbl[], "array"=w1899:dbl[], "array"=w1898:dbl[], "array"=w1897:dbl[], "array"=w1896:dbl[], "array"=w1895:dbl[])
                                n656 = local write "Channel Graph 2"(w1909) -> ()
                                n657 = local write "Channel Graph 3"(w1908) -> ()
                                n658 = local write "Channel Graph 0"(w1911) -> ()
                                n659 = local write "Channel Graph 1"(w1910) -> ()
                                n660 = Insert Into Array(array=w1901, new element=w1910) -> (w1906:dbl[])  [unwired: 1 in]
                                n661 = Insert Into Array(array=w1900, new element=w1909) -> (w1905:dbl[])  [unwired: 1 in]
                                n662 = Insert Into Array(array=w1902, new element=w1911) -> (w1907:dbl[])  [unwired: 1 in]
                                n663 = Insert Into Array(array=w1899, new element=w1908) -> (w1904:dbl[])  [unwired: 1 in]
                                n664 = local write "Channel Graph Cumulative 1"(w1906) -> ()
                                n665 = local write "Channel Graph Cumulative 2"(w1905) -> ()
                                n666 = local write "Channel Graph Cumulative 0"(w1907) -> ()
                                n667 = local write "Channel Graph Cumulative 3"(w1904) -> ()
                                n668 = Bundle("array"=w1907, "array"=w1906, "array"=w1905, "array"=w1904, "array"=w1898, "array"=w1897, "array"=w1896, "array"=w1895) -> (w1894:T7)  [unwired: 1 in]
                              }
                              frame 5 {
                                n669 = disable-structure shown="Enabled" {
                                disable-tunnel: w1947 -> [w1953]
                                disable-tunnel: w1946 -> [w1959]
                                disable-tunnel: [w1954] -> w1944
                                disable-tunnel: [w1955] -> w1943
                                disable-tunnel: [w1956] -> w1942
                                disable-tunnel: [w1957] -> w1941
                                disable-tunnel: [w1958] -> w1940
                                frame Enabled {
                                n670 = call "StandAloneTransient_SingleGraphCreation_DataCollection_Light.vi"("wfm"=w1959, "index"=2, "wfm info"=w1953) -> ("Array"=w1956:dbl[])  [unwired: 8 in]
                                n671 = call "StandAloneTransient_SingleGraphCreation_DataCollection_Light.vi"("wfm"=w1959, "index"=3, "wfm info"=w1953) -> ("Array"=w1957:dbl[])  [unwired: 8 in]
                                n672 = call "StandAloneTransient_SingleGraphCreation_DataCollection_Light.vi"("wfm"=w1959, "index"=0, "wfm info"=w1953) -> ("Array"=w1954:dbl[])  [unwired: 8 in]
                                n673 = call "StandAloneTransient_SingleGraphCreation_DataCollection_Light.vi"("wfm"=w1959, "index"=1, "wfm info"=w1953) -> ("Array"=w1955:dbl[])  [unwired: 8 in]
                                n674 = call "StandAloneTransient_SingleGraphCreation_DataCollection_Light.vi"("wfm"=w1959, "index"=4, "wfm info"=w1953) -> ("Array"=w1958:dbl[])  [unwired: 8 in]
                                }
                                }
                                n675 = Unbundle(w1936) -> ("array"=w1935:dbl[], "array"=w1934:dbl[], "array"=w1933:dbl[], "array"=w1932:dbl[], "array"=w1931:dbl[], "array"=w1928:dbl[], "array"=w1927:dbl[], "array"=w1926:dbl[])
                                n676 = local write "Channel Graph 1"(w1943) -> ()
                                n677 = local write "Channel Graph 3"(w1941) -> ()
                                n678 = local write "Channel Graph 4"(w1940) -> ()
                                n679 = local write "Channel Graph 0"(w1944) -> ()
                                n680 = local write "Channel Graph 2"(w1942) -> ()
                                n681 = Insert Into Array(array=w1933, new element=w1942) -> (w1937:dbl[])  [unwired: 1 in]
                                n682 = Insert Into Array(array=w1932, new element=w1941) -> (w1930:dbl[])  [unwired: 1 in]
                                n683 = Insert Into Array(array=w1935, new element=w1944) -> (w1939:dbl[])  [unwired: 1 in]
                                n684 = Insert Into Array(array=w1934, new element=w1943) -> (w1938:dbl[])  [unwired: 1 in]
                                n685 = Insert Into Array(array=w1931, new element=w1940) -> (w1929:dbl[])  [unwired: 1 in]
                                n686 = local write "Channel Graph Cumulative 2"(w1937) -> ()
                                n687 = local write "Channel Graph Cumulative 3"(w1930) -> ()
                                n688 = local write "Channel Graph Cumulative 0"(w1939) -> ()
                                n689 = local write "Channel Graph Cumulative 1"(w1938) -> ()
                                n690 = local write "Channel Graph Cumulative 4"(w1929) -> ()
                                n691 = Bundle("array"=w1939, "array"=w1938, "array"=w1937, "array"=w1930, "array"=w1929, "array"=w1928, "array"=w1927, "array"=w1926) -> (w1925:T7)  [unwired: 1 in]
                              }
                              frame 6 {
                                n692 = disable-structure shown="Enabled" {
                                disable-tunnel: w1984 -> [w1998]
                                disable-tunnel: w1983 -> [w1996]
                                disable-tunnel: [w1990] -> w1981
                                disable-tunnel: [w1989] -> w1980
                                disable-tunnel: [w1988] -> w1979
                                disable-tunnel: [w1987] -> w1978
                                disable-tunnel: [w1986] -> w1977
                                disable-tunnel: [w1985] -> w1976
                                frame Enabled {
                                n693 = call "StandAloneTransient_SingleGraphCreation_DataCollection_Light.vi"("wfm"=w1998, "index"=2, "wfm info"=w1996) -> ("Array"=w1988:dbl[])  [unwired: 8 in]
                                n694 = call "StandAloneTransient_SingleGraphCreation_DataCollection_Light.vi"("wfm"=w1998, "index"=3, "wfm info"=w1996) -> ("Array"=w1987:dbl[])  [unwired: 8 in]
                                n695 = call "StandAloneTransient_SingleGraphCreation_DataCollection_Light.vi"("wfm"=w1998, "index"=0, "wfm info"=w1996) -> ("Array"=w1990:dbl[])  [unwired: 8 in]
                                n696 = call "StandAloneTransient_SingleGraphCreation_DataCollection_Light.vi"("wfm"=w1998, "index"=1, "wfm info"=w1996) -> ("Array"=w1989:dbl[])  [unwired: 8 in]
                                n697 = call "StandAloneTransient_SingleGraphCreation_DataCollection_Light.vi"("wfm"=w1998, "index"=4, "wfm info"=w1996) -> ("Array"=w1986:dbl[])  [unwired: 8 in]
                                n698 = call "StandAloneTransient_SingleGraphCreation_DataCollection_Light.vi"("wfm"=w1998, "index"=5, "wfm info"=w1996) -> ("Array"=w1985:dbl[])  [unwired: 8 in]
                                }
                                }
                                n699 = Unbundle(w1969) -> ("array"=w1968:dbl[], "array"=w1967:dbl[], "array"=w1966:dbl[], "array"=w1965:dbl[], "array"=w1964:dbl[], "array"=w1963:dbl[], "array"=w1961:dbl[], "array"=w1962:dbl[])
                                n700 = local write "Channel Graph 1"(w1980) -> ()
                                n701 = local write "Channel Graph 4"(w1977) -> ()
                                n702 = local write "Channel Graph 3"(w1978) -> ()
                                n703 = local write "Channel Graph 5"(w1976) -> ()
                                n704 = local write "Channel Graph 0"(w1981) -> ()
                                n705 = local write "Channel Graph 2"(w1979) -> ()
                                n706 = Insert Into Array(array=w1966, new element=w1979) -> (w1973:dbl[])  [unwired: 1 in]
                                n707 = Insert Into Array(array=w1965, new element=w1978) -> (w1972:dbl[])  [unwired: 1 in]
                                n708 = Insert Into Array(array=w1968, new element=w1981) -> (w1975:dbl[])  [unwired: 1 in]
                                n709 = Insert Into Array(array=w1967, new element=w1980) -> (w1974:dbl[])  [unwired: 1 in]
                                n710 = Insert Into Array(array=w1964, new element=w1977) -> (w1971:dbl[])  [unwired: 1 in]
                                n711 = Insert Into Array(array=w1963, new element=w1976) -> (w1970:dbl[])  [unwired: 1 in]
                                n712 = local write "Channel Graph Cumulative 2"(w1973) -> ()
                                n713 = local write "Channel Graph Cumulative 3"(w1972) -> ()
                                n714 = local write "Channel Graph Cumulative 0"(w1975) -> ()
                                n715 = local write "Channel Graph Cumulative 1"(w1974) -> ()
                                n716 = local write "Channel Graph Cumulative 4"(w1971) -> ()
                                n717 = local write "Channel Graph Cumulative 5"(w1970) -> ()
                                n718 = Bundle("array"=w1975, "array"=w1974, "array"=w1973, "array"=w1972, "array"=w1971, "array"=w1970, "array"=w1961, "array"=w1962) -> (w1960:T7)  [unwired: 1 in]
                              }
                              frame 7 {
                                n719 = disable-structure shown="Enabled" {
                                disable-tunnel: w2025 -> [w2040]
                                disable-tunnel: w2024 -> [w2039]
                                disable-tunnel: [w2041] -> w2022
                                disable-tunnel: [w2038] -> w2021
                                disable-tunnel: [w2037] -> w2020
                                disable-tunnel: [w2036] -> w2019
                                disable-tunnel: [w2035] -> w2018
                                disable-tunnel: [w2034] -> w2017
                                disable-tunnel: [w2033] -> w2016
                                frame Enabled {
                                n720 = call "StandAloneTransient_SingleGraphCreation_DataCollection_Light.vi"("wfm"=w2039, "index"=3, "wfm info"=w2040) -> ("Array"=w2036:dbl[])  [unwired: 8 in]
                                n721 = call "StandAloneTransient_SingleGraphCreation_DataCollection_Light.vi"("wfm"=w2039, "index"=4, "wfm info"=w2040) -> ("Array"=w2035:dbl[])  [unwired: 8 in]
                                n722 = call "StandAloneTransient_SingleGraphCreation_DataCollection_Light.vi"("wfm"=w2039, "index"=0, "wfm info"=w2040) -> ("Array"=w2041:dbl[])  [unwired: 8 in]
                                n723 = call "StandAloneTransient_SingleGraphCreation_DataCollection_Light.vi"("wfm"=w2039, "index"=1, "wfm info"=w2040) -> ("Array"=w2038:dbl[])  [unwired: 8 in]
                                n724 = call "StandAloneTransient_SingleGraphCreation_DataCollection_Light.vi"("wfm"=w2039, "index"=2, "wfm info"=w2040) -> ("Array"=w2037:dbl[])  [unwired: 8 in]
                                n725 = call "StandAloneTransient_SingleGraphCreation_DataCollection_Light.vi"("wfm"=w2039, "index"=5, "wfm info"=w2040) -> ("Array"=w2034:dbl[])  [unwired: 8 in]
                                n726 = call "StandAloneTransient_SingleGraphCreation_DataCollection_Light.vi"("wfm"=w2039, "index"=6, "wfm info"=w2040) -> ("Array"=w2033:dbl[])  [unwired: 8 in]
                                }
                                }
                                n727 = Unbundle(w2007) -> ("array"=w2006:dbl[], "array"=w2005:dbl[], "array"=w2004:dbl[], "array"=w2003:dbl[], "array"=w2002:dbl[], "array"=w2001:dbl[], "array"=w2000:dbl[], "array"=w1999:dbl[])
                                n728 = local write "Channel Graph 2"(w2020) -> ()
                                n729 = local write "Channel Graph 1"(w2021) -> ()
                                n730 = local write "Channel Graph 5"(w2017) -> ()
                                n731 = local write "Channel Graph 6"(w2016) -> ()
                                n732 = local write "Channel Graph 0"(w2022) -> ()
                                n733 = local write "Channel Graph 3"(w2019) -> ()
                                n734 = local write "Channel Graph 4"(w2018) -> ()
                                n735 = Insert Into Array(array=w2003, new element=w2019) -> (w2011:dbl[])  [unwired: 1 in]
                                n736 = Insert Into Array(array=w2002, new element=w2018) -> (w2010:dbl[])  [unwired: 1 in]
                                n737 = Insert Into Array(array=w2006, new element=w2022) -> (w2015:dbl[])  [unwired: 1 in]
                                n738 = Insert Into Array(array=w2005, new element=w2021) -> (w2013:dbl[])  [unwired: 1 in]
                                n739 = Insert Into Array(array=w2004, new element=w2020) -> (w2012:dbl[])  [unwired: 1 in]
                                n740 = Insert Into Array(array=w2001, new element=w2017) -> (w2009:dbl[])  [unwired: 1 in]
                                n741 = Insert Into Array(array=w2000, new element=w2016) -> (w2008:dbl[])  [unwired: 1 in]
                                n742 = local write "Channel Graph Cumulative 3"(w2011) -> ()
                                n743 = local write "Channel Graph Cumulative 4"(w2010) -> ()
                                n744 = local write "Channel Graph Cumulative 0"(w2015) -> ()
                                n745 = local write "Channel Graph Cumulative 1"(w2013) -> ()
                                n746 = local write "Channel Graph Cumulative 2"(w2012) -> ()
                                n747 = local write "Channel Graph Cumulative 5"(w2009) -> ()
                                n748 = local write "Channel Graph Cumulative 6"(w2008) -> ()
                                n749 = Bundle("array"=w2015, "array"=w2013, "array"=w2012, "array"=w2011, "array"=w2010, "array"=w2009, "array"=w2008, "array"=w1999) -> (w2014:T7)  [unwired: 1 in]
                              }
                              frame 8 {
                                n750 = disable-structure shown="Enabled" {
                                disable-tunnel: w2070 -> [w2087]
                                disable-tunnel: w2069 -> [w2088]
                                disable-tunnel: [w2071] -> w2067
                                disable-tunnel: [w2072] -> w2066
                                disable-tunnel: [w2073] -> w2065
                                disable-tunnel: [w2074] -> w2064
                                disable-tunnel: [w2075] -> w2063
                                disable-tunnel: [w2076] -> w2062
                                disable-tunnel: [w2077] -> w2061
                                disable-tunnel: [w2078] -> w2060
                                frame Enabled {
                                n751 = call "StandAloneTransient_SingleGraphCreation_DataCollection_Light.vi"("wfm"=w2088, "index"=3, "wfm info"=w2087) -> ("Array"=w2074:dbl[])  [unwired: 8 in]
                                n752 = call "StandAloneTransient_SingleGraphCreation_DataCollection_Light.vi"("wfm"=w2088, "index"=4, "wfm info"=w2087) -> ("Array"=w2075:dbl[])  [unwired: 8 in]
                                n753 = call "StandAloneTransient_SingleGraphCreation_DataCollection_Light.vi"("wfm"=w2088, "index"=0, "wfm info"=w2087) -> ("Array"=w2071:dbl[])  [unwired: 8 in]
                                n754 = call "StandAloneTransient_SingleGraphCreation_DataCollection_Light.vi"("wfm"=w2088, "index"=1, "wfm info"=w2087) -> ("Array"=w2072:dbl[])  [unwired: 8 in]
                                n755 = call "StandAloneTransient_SingleGraphCreation_DataCollection_Light.vi"("wfm"=w2088, "index"=2, "wfm info"=w2087) -> ("Array"=w2073:dbl[])  [unwired: 8 in]
                                n756 = call "StandAloneTransient_SingleGraphCreation_DataCollection_Light.vi"("wfm"=w2088, "index"=5, "wfm info"=w2087) -> ("Array"=w2076:dbl[])  [unwired: 8 in]
                                n757 = call "StandAloneTransient_SingleGraphCreation_DataCollection_Light.vi"("wfm"=w2088, "index"=6, "wfm info"=w2087) -> ("Array"=w2077:dbl[])  [unwired: 8 in]
                                n758 = call "StandAloneTransient_SingleGraphCreation_DataCollection_Light.vi"("wfm"=w2088, "index"=7, "wfm info"=w2087) -> ("Array"=w2078:dbl[])  [unwired: 8 in]
                                }
                                }
                                n759 = Unbundle(w2050) -> ("array"=w2049:dbl[], "array"=w2048:dbl[], "array"=w2047:dbl[], "array"=w2046:dbl[], "array"=w2045:dbl[], "array"=w2044:dbl[], "array"=w2043:dbl[], "array"=w2042:dbl[])
                                n760 = local write "Channel Graph 2"(w2065) -> ()
                                n761 = local write "Channel Graph 5"(w2062) -> ()
                                n762 = local write "Channel Graph 1"(w2066) -> ()
                                n763 = local write "Channel Graph 6"(w2061) -> ()
                                n764 = local write "Channel Graph 7"(w2060) -> ()
                                n765 = local write "Channel Graph 0"(w2067) -> ()
                                n766 = local write "Channel Graph 3"(w2064) -> ()
                                n767 = local write "Channel Graph 4"(w2063) -> ()
                                n768 = Insert Into Array(array=w2046, new element=w2064) -> (w2056:dbl[])  [unwired: 1 in]
                                n769 = Insert Into Array(array=w2045, new element=w2063) -> (w2055:dbl[])  [unwired: 1 in]
                                n770 = Insert Into Array(array=w2049, new element=w2067) -> (w2059:dbl[])  [unwired: 1 in]
                                n771 = Insert Into Array(array=w2048, new element=w2066) -> (w2058:dbl[])  [unwired: 1 in]
                                n772 = Insert Into Array(array=w2047, new element=w2065) -> (w2057:dbl[])  [unwired: 1 in]
                                n773 = Insert Into Array(array=w2044, new element=w2062) -> (w2054:dbl[])  [unwired: 1 in]
                                n774 = Insert Into Array(array=w2043, new element=w2061) -> (w2052:dbl[])  [unwired: 1 in]
                                n775 = Insert Into Array(array=w2042, new element=w2060) -> (w2051:dbl[])  [unwired: 1 in]
                                n776 = local write "Channel Graph Cumulative 3"(w2056) -> ()
                                n777 = local write "Channel Graph Cumulative 4"(w2055) -> ()
                                n778 = local write "Channel Graph Cumulative 0"(w2059) -> ()
                                n779 = local write "Channel Graph Cumulative 1"(w2058) -> ()
                                n780 = local write "Channel Graph Cumulative 2"(w2057) -> ()
                                n781 = local write "Channel Graph Cumulative 5"(w2054) -> ()
                                n782 = local write "Channel Graph Cumulative 6"(w2052) -> ()
                                n783 = local write "Channel Graph Cumulative 7"(w2051) -> ()
                                n784 = Bundle("array"=w2059, "array"=w2058, "array"=w2057, "array"=w2056, "array"=w2055, "array"=w2054, "array"=w2052, "array"=w2051) -> (w2053:T7)  [unwired: 1 in]
                              }
                              frame 9.. {
                              }
                            }
                          }
                        }
                      }
                    }
                  }
                }
                "Collecting Data" <- w1497
              }
              frame "HOLDBY", Default {
                n785 = case shown="False" w2100 {
                  tunnel: [w2105 "INITIALIZE"] -> w2103
                  tunnel: w2099 -> [w2104 _]
                  frame False {
                    n786 = case shown="False" w2104 {
                      tunnel: ["HOLDBY" "CONFIGSCOPE"] -> w2105
                      frame False {
                      }
                      frame True {
                      }
                    }
                  }
                  frame True {
                  }
                }
                "RECORDING DATA" <- w2100
                "INITIALIZED" <- w2100
              }
            }
            "Number Of Channels" <- w990
            "Num Loop 4 Reset Graph" <- w984
            n787 = local read "FINISH PROGRAM"() -> (w1022:bool)
            "Min. Sample Rate IND" <- "Min. Sample Rate"
            "channels IND" <- "channels"
            "Vertical Range (V) IND" <- "Vertical Range (V)"
          }
          n788 = Release Queue(queue=w398, error in (no error)=w414) -> (error out=w413:errorcluster)  [unwired: 1 in, 2 out]
          n789 = call <instrlib>:"niScope Close.vi"("instrument handle"=w419, "error in"=w413) -> ("error out"=w415:errorcluster)  [unwired: 13 in]
          n790 = VISA Close(VISA resource name=w387, error in (no error)=w389) -> (error out=w388:errorcluster)
          n791 = Merge Errors(w388) -> (w390:errorcluster)
          n792 = Merge Errors(w416, w415, w390) -> (w386:errorcluster)
        }
      }
      n793 = call <vilib>:"Simple Error Handler.vi"("error in (no error)"=w371) -> ()  [unwired: 4 in, 5 out]
    }
    frame Disabled {
    }
  }
